vi "MoD Main-Optimize - Raman PK.vi"() -> ()   [LabVIEW 2015]
uses:
  <vilib>/silver_ctls/ArrayMatrixCluster/Real Matrix NI_Silver.ctl
  <vilib>/ni845x/ni845x.llb/ni845xControl.ctl
  <vilib>/MakerHub/LINX/Public/Peripherals/Analog/Analog Read 1 Chan.vi
  <vilib>/MakerHub/LINX/Public/Peripherals/Analog/Analog Read N Chans.vi
  <vilib>/MakerHub/LINX/Private/Local IO/LinxAnalogRead.vi
  <vilib>/MakerHub/LINX/Public/Utilities/Check Channel.vi
  <vilib>/addons/control/pid/pid.llb/PID Control Input Filter (DBL).vi
  <vilib>/MakerHub/LINX/Private/Utilties/Generate Error.vi
  <vilib>/addons/control/pid/autopid.llb/PID Online Autotuning (Relay Feedback).vi
  <vilib>/Analysis/Matrix/Numeric/Conversions/Array To Matrix - RA2.vi
  <vilib>/ni845x/ni845x.llb/NI-845x Close Device Reference.vi
  <vilib>/addons/control/pid/NI_PID_autopid.lvlib
  <vilib>/addons/control/pid/NI_PID_pid.lvlib
  <vilib>/Analysis/Matrix/NI_Matrix.lvlib
  <vilib>/MakerHub/LINX/LMH-LINX.lvlib
  <instrlib>/Harvard Apparatus PHD Ultra Series/Harvard Apparatus PHD Ultra Series.lvlib
panel:
  out "running?":bool=TRUE
  out "new_reactor_volume":bool[](array[boolean])
  out "new_reactor_length":bool[](array[boolean])
  out "Phase_Sensor_voltage":dbl
  out "P_tot":dbl
  out "pause for ms":bool=TRUE
  out "stop_xl_write":bool=TRUE
  out "Num_exp_till_pause":i32
  out "Syringe_pump?":bool=TRUE
  out "System Error":bool=TRUE
  out "error out":errorcluster
  out "Pump setpoint(ul/min) 6":dbl format="%#_13g"
  out "Pump setpoint(ul/min) 5":dbl format="%#_13g"
  out "Pump setpoint(ul/min) 4":dbl format="%#_13g"
  out "Pump setpoint(ul/min) 3":dbl format="%#_13g"
  out "Pump setpoint(ul/min) 2":dbl format="%#_13g"
  out "Pump setpoint(ul/min) 1":dbl format="%#_13g"
  out "Volume (ul) 5":dbl format="%#_13g"
  out "Volume (ul) 4":dbl format="%#_13g"
  out "Volume (ul) 3":dbl format="%#_13g"
  out "Volume (ul) 2":dbl format="%#_13g"
  out "Volume (ul) 1":dbl format="%#_13g"
  in  "tau 5":dbl format="%#_13g"
  out "tau 4":dbl format="%#_13g"
  out "tau 3":dbl format="%#_13g"
  out "tau 2":dbl format="%#_13g"
  out "tau 1":dbl format="%#_13g"
  out "Reactor Length":dbl format="%#_13g"
  out "Flowrate Sensor 2":dbl format="%#_13g"
  out "Flowrate Sensor 1":dbl format="%#_13g"
  out "Pressure 2":dbl format="%#_13g"
  out "Pressure 1":dbl format="%#_13g"
  out "Temperature Control 5":bool=TRUE
  out "Temperature Control 4":bool=TRUE
  out "Temperature Control 3":bool=TRUE
  out "Temperature Control 2":bool=TRUE
  out "Temperature Control 1":bool=TRUE
  out "Temperature SP 5":dbl format="%#_g'C"
  out "Temperature SP 4":dbl format="%#_g'C"
  out "Temperature SP 3":dbl format="%#_g'C"
  out "Temperature SP 2":dbl format="%#_g'C"
  out "Temperature SP 1":dbl format="%#_g'C"
  in  "Bay Temperature 5":dbl
  in  "SSR Duration 5":dbl
  in  "SSR Duration 4":dbl
  in  "SSR Duration 3":dbl
  in  "SSR Duration 2":dbl
  in  "SSR Duration 1":dbl
  in  "Total Product Amount":dbl=1.0 format="%#_gml"
  out "Setup Error":bool=TRUE
  out "Error Message":string
  out "ID CTR":i32
  in  "Tab Control":T1(tab)
  out "Reagent pic 5":picture
  in  "reagent name 5":string
  out "Reagent Pic 4":picture
  in  "reagent name 4":string=" 2,5-hexanedione"
  out "Reagent Pic 3":picture
  in  "reagent  name 3":string
  in  "Product name":string
  in  "reagent name 1":string="2,5-hexanedione"
  out "Reagent Pic 1":picture
  in  "Vr5":dbl format="%#_guL"
  in  "Vr4":dbl format="%#_guL"
  in  "Vr3":dbl format="%#_guL"
  in  "Vr2":dbl format="%#_guL"
  in  "Vr1":dbl format="%#_guL"
  in  "System decide help Button":bool
  in  "Reaction Scheme Confirm":bool
  in  "Synthesis Route Array":string[][](array[string])=[["Hexanedione", "1", "PhB(OH)2", "", "", ""], ["ethanolamine", "1", "-", "-", "-", "-"], ["", "", "-", "-", "-", "-"], ["", "", "-", "-", "-", "-"], ["", "", "-", "-", "-", "-"], ["", "", "-", "-", "-", "-"]]
  in  "System decide help Button 2":bool
  out "Setup Confirm":bool=TRUE
  in  "BAY 1":u16(ring) items=["               Bypass", "         Heated Reactor", "    Small Heated Reator", "         Cooled Reactor", "      Packed Bed Reactor", "          Photo Reactor", "             Separator"]
  in  "BAY 5":u16(ring) items=["               Bypass", "         Heated Reactor", "    Small Heated Reactor", "         Cooled Reactor", "     Packed Bed Reactor", "         Photo Reactor", "             Separator"]
  in  "BAY 4":u16(ring) items=["                Bypass", "         Heated Reactor", "    Small Heated Reactor", "         Cooled Reactor", "     Packed Bed Reactor", "         Photo Reactor", "             Separator"]
  in  "BAY 3":u16(ring)=2 items=["               Bypass", "         Heated Reactor", "    Small Heated Reactor", "         Cooled Reactor", "     Packed Bed Reactor", "          Photo Reactor", "             Separator"]
  in  "BAY 2":u16(ring) items=["               Bypass", "         Heated Reactor", "    Small Heated Reactor", "         Cooled Reactor", "      Packed Bed Reactor", "          Photo Reactor", "             Separator"]
  out "Reagent Pic 2":picture
  out "Product Pic":picture
  in  "reagent name 2":string="ethanolamine"
  in  "reagent name 6":string
  out "Reagent Pic 6":picture
  in  "System Parameters Help Button":bool
  out "Setup Confirm 2":bool
  in  "System Parameters Confirm Button":bool
  in  "Bay Parameters":T2={"Bay 1 "={"Pump 1 Flowrate"=0.0, "optimize_temp"=FALSE, "optimize_tau"=FALSE, "Run at set flowrate"=FALSE, "Pump 2 Flowrate"=0.0, "Temperature Params"=[40.0, 100.0, 100.0], "pump params 1"=[57.0, 122.0, 325.0], "pump params 2"=[57.0, 122.0, 325.0], "Temperature"=0.0, "Run at set temperature"=FALSE}, "Bay 2 "={"Pump 3 Flowrate"=0.0, "optimize_temp"=FALSE, "optimize_tau"=FALSE, "Run at set flowrate"=FALSE, "Temperature Params"=[40.0, 100.0, 100.0], "Resisdence time params"=[1.0, 5.0, 650.0], "pump_at_ratio"=FALSE, "pump_num_ratio"=4.0, "Temperature"=0.0, "Run at set temperature"=FALSE}, "Bay 3 "={"Pump 4 Flowrate"=100.0, "optimize_temp"=TRUE, "optimize_tau"=TRUE, "Run at set flowrate"=FALSE, "Temperature Params"=[40.0, 80.0, 100.0], "Resisdence time params"=[40.0, 401.0, 0.0], "pump_at_ratio"=FALSE, "pump_num_ratio"=0.05, "Temperature "=0.0, "Run at set temperature"=FALSE}, "Bay 4 "={"Pump 5 Flowrate"=40.0, "Run at set flowrate"=FALSE, "optimize_temp"=FALSE, "optimize_tau"=FALSE, "Resisdence time params"=[40.6, 406.0, 225.0], "Temperature Params"=[40.0, 100.0, 80.0], "pump_at_ratio"=FALSE, "pump_num_ratio"=1.0, "Temperature"=0.0, "Run at set temperature"=FALSE}, "Bay 5 "={"Pump 6 Flowrate"=0.0, "Run at set flowrate"=FALSE, "optimize_temp"=FALSE, "optimize_tau"=FALSE, "Resisdence time params"=[7.62, 114.27, 0.0], "Temperature Params"=[0.0, 0.0, 0.0], "pump_at_ratio"=FALSE, "pump_num_ratio"=0.5, "Temperature"=0.0, "Run at set temperature"=FALSE}, "Excel File Name"="C:\\Users\\HPLC\\Dropbox (MIT)\\MoD Files\\Data\\PK_Raman08302017", "Raman File Name"="\\\\Desktop-ld0eu12\\c\\Data\\MoD\\Paal_Knorr", "Matlab File"="C:\\Users\\HPLC\\Dropbox (MIT)\\MoD Files\\Data\\PK_Raman08302017_1", "Syringe for Pump 2?"=FALSE, "Num_conditons_per_wait"=2.0, "Continue from previous optimization?"=FALSE, "Total Number of Experiments 2"=12.0, "Hplc Wait time(min)"=8.0, "increas_decrease_hplc_peak"=TRUE, "Internal Standard?"=TRUE, "ISTD start"=3.0, "ISTD end"=4.0, "hplc_start"=6.0, "hplc_end"=7.0, "throughput_yield"=FALSE} {"Hplc Wait time(min)" format="%#_13g"; "Bay 5"."Temperature Params" format="%#_g'C"; "Bay 4"."Temperature Params" format="%#_g'C"; "Bay 3"."Temperature Params" format="%#_g'C"; "Bay 2"."Temperature Params" format="%#_g'C"; "Bay 1"."Temperature Params" format="%#_g'C"}
  out "System Confirm Not Clicked":string
  out "best_exp_num":dbl=1.0
  out "temperature_best":dbl[](array[numeric])
  out "Flowrates(ul/min)_best":dbl[](array[numeric])
  out "System Status":u16(ring)=2 caption="Sy" items=["System  Error", "System Running", "System Standby"]
  out "Current Experiment":dbl=1.0
  out "Total Number of Experiments":dbl=33.0
  out "Phase Sensor Chart":T3(graph)
  out "HPLC Analysis":bool
  out "Equlibrating Temperature":bool
  out "Flushing System":bool
  out "Calculate condition":bool
  out "Temperature 5":dbl format="%#_g'C"
  out "Temperature 4":dbl format="%#_g'C"
  out "Temperature 3":dbl format="%#_g'C"
  out "Temperature 2":dbl format="%#_g'C"
  out "Temperature 1":dbl format="%#_g'C"
  out "Flowrate Chart":T4(graph)
  out "Teperature Chart":T3(graph)
  out "Pump Setpoints Chart":T3(graph)
  out "Pressure Chart":T3(graph)
  out "Optimization_loop_index":i32
  out "curr_wait_time":dbl
  out "total_flush_time":dbl
  out "Temp SS? 5":bool=TRUE
  out "Temp SS? 4":bool=TRUE
  out "Temp SS? 3":bool=TRUE
  out "Temp SS? 2":bool=TRUE
  out "Temp SS? 1":bool=TRUE
  out "System Flushed?":bool
  out "stop_button clicked":bool
  out "experiment history":T5
  in  "Number of System Flushes per condtion":dbl=2.5
  in  "calculate volume 3":bool=TRUE
  in  "calculate volume 2":bool=TRUE
  in  "calculate volume 1":bool=TRUE
  in  "calculate volume 4":bool
  in  "calculate volume 5":bool
  in  "Extra system dead volume":dbl format="%#_gul"
  in  "new reactor length? 1":bool
  in  "tube_length(in)":dbl[](array[numeric])=[188.0, 188.0, 10.0, 10.0, 10.0]
  out "Pause Before Analysis":bool
  out "Chiller COMM Port":bool
  out "Arduino COMM Port 2":bool
  out "Temperature Sensor COMM Port":bool
  out "Flow Rate":bool
  out "Pressure":bool
  out "Pump COMM Port":bool
  in  "COMM Port :: Milligat Pumps":refnum<visa-resource-name>="COM10"
  in  "Arduino COMM Port":refnum<visa-resource-name>="COM3"
  in  "Sample Valve COMM::Port":refnum<visa-resource-name>="COM4"
  in  "COMM Port:: Harvard Syringe Pump":refnum<visa-resource-name>="COM5"
  in  "tube_id(in)":enum16{".01", ".02", ".03", ".04"}[](array[ring])=[enum.".03", enum.".03", enum.".03", enum.".03", enum.".03"]
  out "Total System Resisdence Time(min)":dbl
  in  "Debug_run_button":bool
  in  "new reactor length? 2":bool
  in  "new reactor length? 3":bool
  in  "new reactor length? 4":bool
  in  "new reactor length? 5":bool
  in  "IR Sensor Device":T6="USB0::0x3923::0x7514::01B3FF21::RAW"
  out "Stop":bool=TRUE
  in  "Run_Stop_cluster":T7
  # "Molecules on Demand"
  # "Synthetic Route"
  # "5"
  # "6"
  # "4"
  # "Product"
  # "1"
  # "2"
  # "3"
  # "Reagent List"
  # "Concentration(M)"
  # "Molecule"
  # "1"
  # "1"
  # "2"
  # "2"
  # "3"
  # "3"
  # "4"
  # "4"
  # "5"
  # "6"
  # "5"
  # "6"
  # "Product"
  # "Reactor Volume:"
  # "Optimization Parameters"
  # "Pause after"
  # "Experiments"
  # "Optimize for"
  # "to"
  # "of HPLC Peak from"
  # "from"
  # "to"
  # "min"
  # "min"
  # "HPLC runtime"
  # "# Iterations"
  # "Reporting"
  # "Excel Output File Name"
  # "Raman File Path"
  # "MATLAB File Path"
  # "Temperature"
  # "Flowrate(ul/min)"
  # "Lower Bound"
  # "Upper Bound"
  # "Optimize?"
  # "-or-"
  # "Run at"
  # "times incoming flow"
  # "Setpoint"
  # "Temperature"
  # "Flowrate(ul/min)"
  # "Lower Bound"
  # "Upper Bound"
  # "Optimize?"
  # "-or-"
  # "Run at"
  # "times incoming flow"
  # "Setpoint"
  # "Temperature"
  # "Flowrate(ul/min)"
  # "Lower Bound"
  # "Upper Bound"
  # "Optimize?"
  # "-or-"
  # "Run at"
  # "times incoming flow"
  # "Setpoint"
  # "Temperature"
  # "Flowrate 3 (ul/min)"
  # "Lower Bound"
  # "Upper Bound"
  # "Optimize?"
  # "-or-"
  # "Run at"
  # "times incoming flow"
  # "Setpoint"
  # "Temperature"
  # "Flowrate 1(ul/min)"
  # "Flowrate 2(ul/min)"
  # "Lower Bound"
  # "Upper Bound"
  # "Optimize?"
  # "Setpoint"
  # "Pressure (psi)"
  # "System Status"
  # "Temperature('C)"
  # "BAY"
  # "1"
  # "2"
  # "3"
  # "4"
  # "5"
  # "Pump Flowrate Setpoint(ul/min)"
  # "Flowrate (ul/min)"
  # "Phase Sensor"
  # "Current Experiment"
  # "Temperature('C)"
  # "Flowrate(ul/min)"
  # "Exp"
  # "Current Best Condition"
  # "Time to reach steady state:"
  # "Current Wait Time:"
  # "Experimental Steps"
  # "Calculated New Conditions"
  # "Steady State"
  # "Analyzed Raman"
  # "Equilibrated Temperature"
  # "Tube Length (cm)"
  # "Bay"
  # "Tube ID (in)"
  # "Calculate Volume"
  # "Use new tube length"
  # "1."
  # "2."
  # "3."
  # "4."
  # "5."
  # "Reactor Lengths\n*Heated Reactor - 188cm * Small Reactor - 99cm * Bypass - 10cm * Separator - *"
  # "All Experimental Data"
  # "P1"
  # "P2"
  # "P3"
  # "P4"
  # "P5"
  # "P6"
  # "T1"
  # "T2"
  # "T3"
  # "T4"
  # "T5"
  # "Obj_fun"
  # "HPLC_Data"
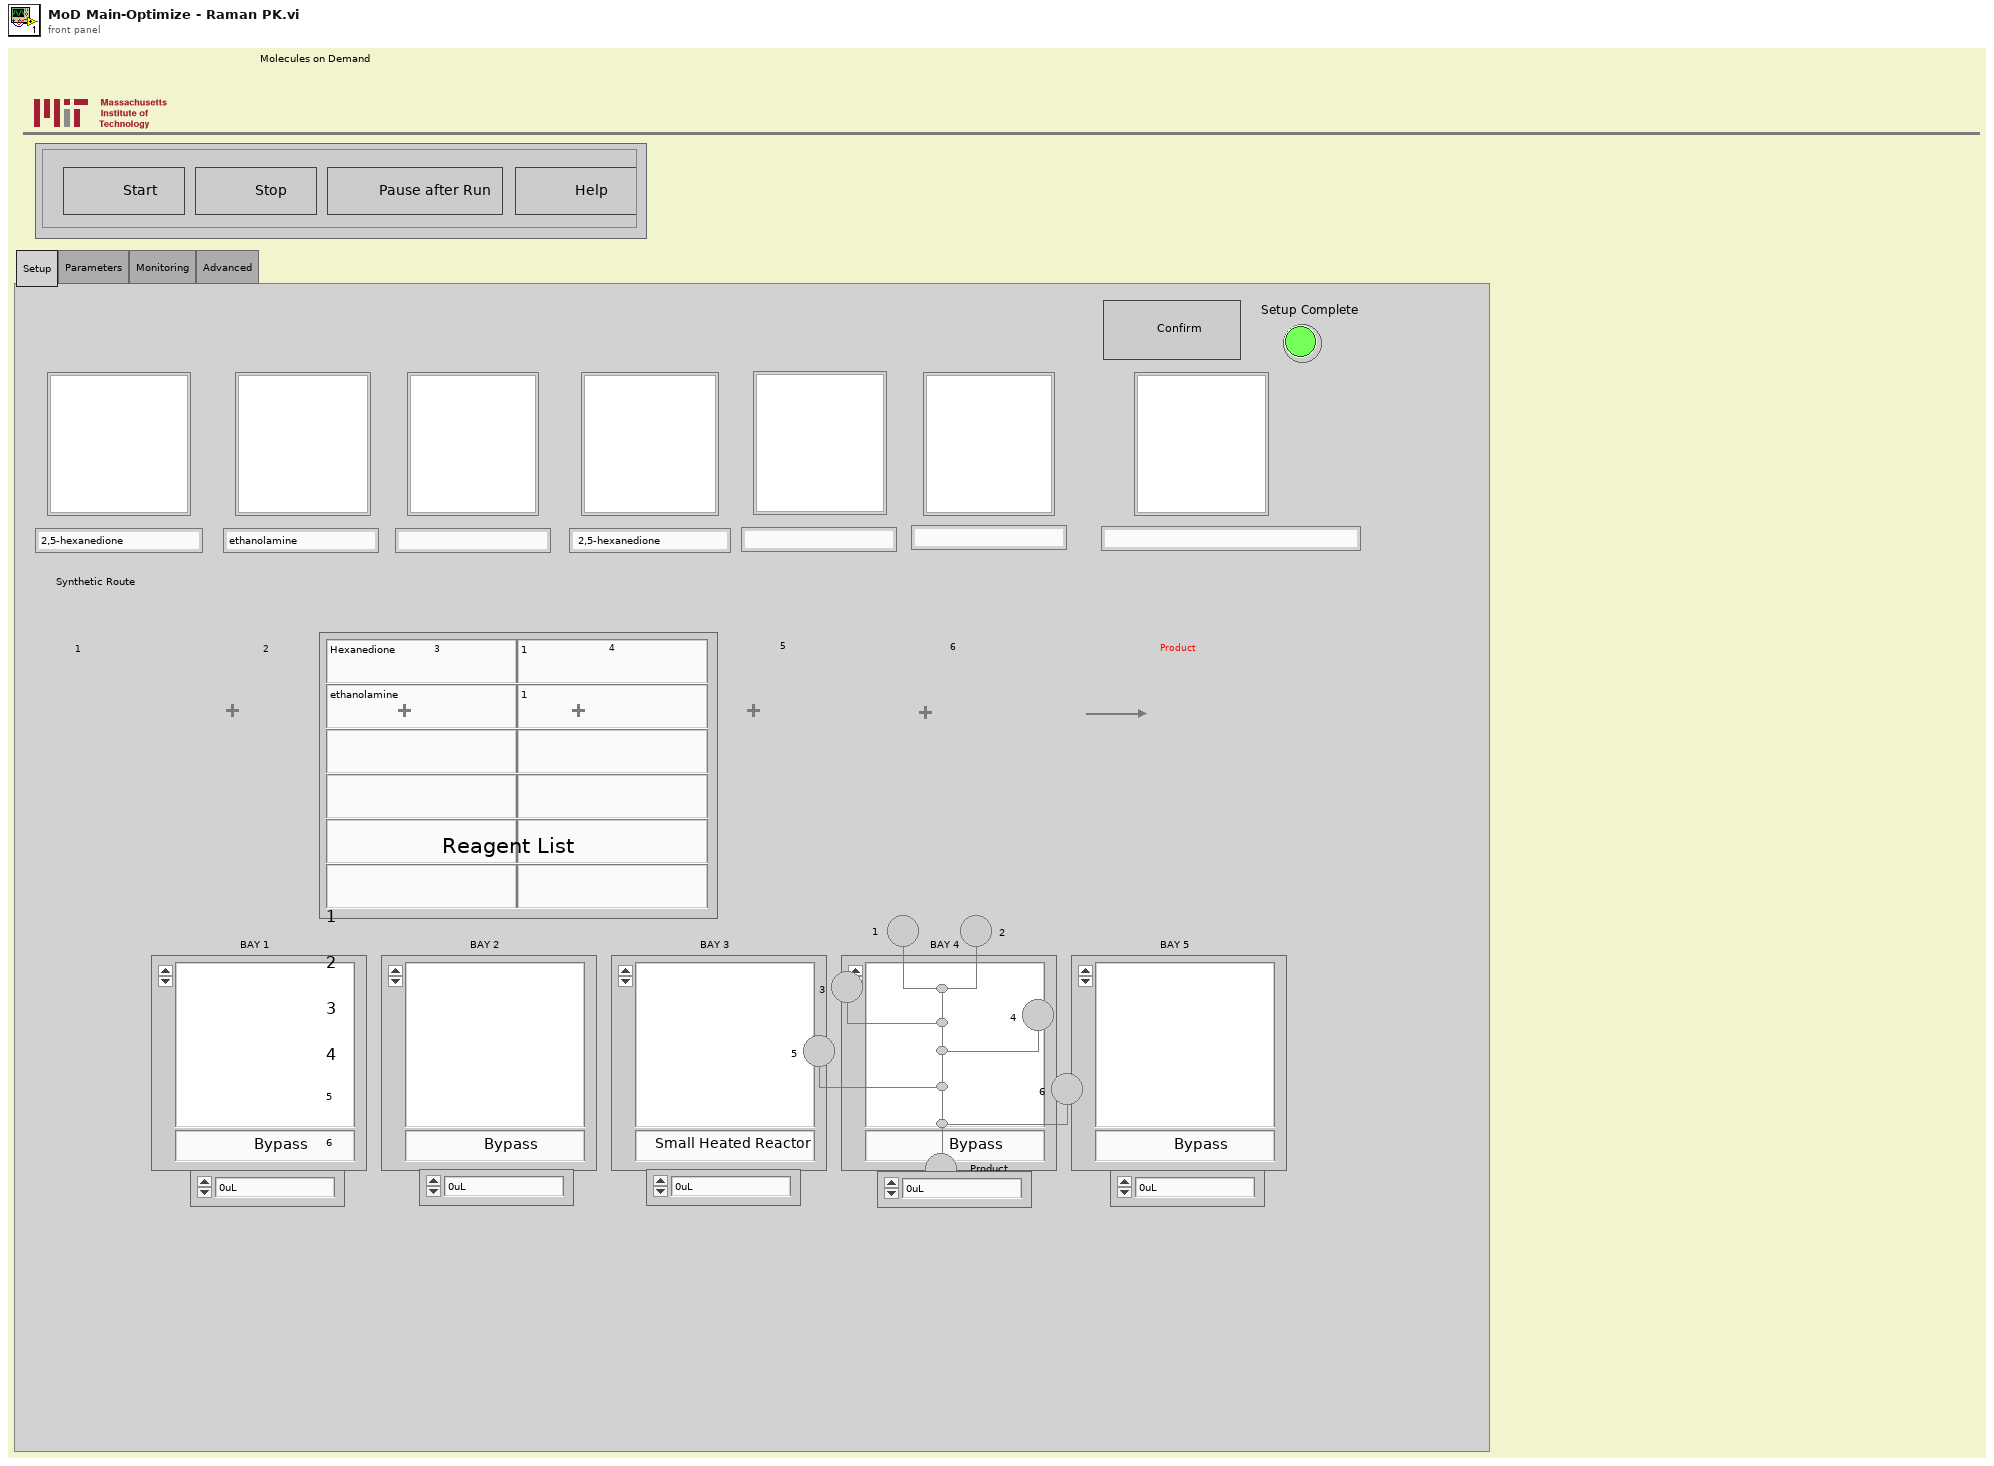
[diagram p1: front panel]
types:
  T1 = enum32{"Setup", "Parameters", "Monitoring", "Advanced"}
  T2 = cluster{"Bay 1 ":cluster{"Pump 1 Flowrate":dbl, "optimize_temp":bool, "optimize_tau":bool, "Run at set flowrate":bool, "Pump 2 Flowrate":dbl, "Temperature Params":dbl[], "pump params 1":dbl[], "pump params 2":dbl[], "Temperature":dbl, "Run at set temperature":bool}, "Bay 2 ":cluster{"Pump 3 Flowrate":dbl, "optimize_temp":bool, "optimize_tau":bool, "Run at set flowrate":bool, "Temperature Params":dbl[], "Resisdence time params":dbl[], "pump_at_ratio":bool, "pump_num_ratio":dbl, "Temperature":dbl, "Run at set temperature":bool}, "Bay 3 ":cluster{"Pump 4 Flowrate":dbl, "optimize_temp":bool, "optimize_tau":bool, "Run at set flowrate":bool, "Temperature Params":dbl[], "Resisdence time params":dbl[], "pump_at_ratio":bool, "pump_num_ratio":dbl, "Temperature ":dbl, "Run at set temperature":bool}, "Bay 4 ":cluster{"Pump 5 Flowrate":dbl, "Run at set flowrate":bool, "optimize_temp":bool, "optimize_tau":bool, "Resisdence time params":dbl[], "Temperature Params":dbl[], "pump_at_ratio":bool, "pump_num_ratio":dbl, "Temperature":dbl, "Run at set temperature":bool}, "Bay 5 ":cluster{"Pump 6 Flowrate":dbl, "Run at set flowrate":bool, "optimize_temp":bool, "optimize_tau":bool, "Resisdence time params":dbl[], "Temperature Params":dbl[], "pump_at_ratio":bool, "pump_num_ratio":dbl, "Temperature":dbl, "Run at set temperature":bool}, "Excel File Name":string, "Raman File Name":string, "Matlab File":string, "Syringe for Pump 2?":bool, "Num_conditons_per_wait":dbl, "Continue from previous optimization?":bool, "Total Number of Experiments 2":dbl, "Hplc Wait time(min)":dbl, "increas_decrease_hplc_peak":bool, "Internal Standard?":bool, "ISTD start":dbl, "ISTD end":dbl, "hplc_start":dbl, "hplc_end":dbl, "throughput_yield":bool}
  T3 = cluster{"[0]":dbl, "[1]":dbl, "[2]":dbl, "[3]":dbl, "[4]":dbl, "[5]":dbl, "[6]":dbl, "[7]":dbl, "[8]":dbl}
  T4 = cluster{"[0]":i32, "[1]":i32, "[2]":i32, "[3]":i32, "[4]":i32, "[5]":i32, "[6]":i32, "[7]":i32, "[8]":i32}
  T5 = typedef "Real Matrix NI_Silver.ctl" = dbl[][]
  T6 = typedef "ni845xControl.ctl" = refnum<k21>
  T7 = cluster{"Stop":bool, "Run":bool, "Stop Run Button":bool, "Help Button":bool}
  T8 = cluster{"Proportional gain Kc":dbl, "Integral time Ti (sec)":dbl, "Derivative time Ti (sec)":dbl}
  T9 = cluster{"type of controller":enum16{"P", "PI", "PID"}, "relay cycles":i32, "relay amplitude":dbl, "control specifications":enum16{"Fast", "Normal", "Slow"}, "PV noise level":dbl}
  T10 = typedef "LMH-LINX.lvlib/LINX Ref.ctl" = cluster{"IO":T11, "Interface":T12, "LINX Device Config":T13}
  T11 = typedef "LMH-LINX.lvlib/Platform.ctl" = enum16{"Remote", "Local"}
  T12 = typedef "LMH-LINX.lvlib/Interface.ctl" = enum16{"Serial", "TCP"}
  T13 = typedef "LMH-LINX.lvlib/Device.lvlib/LINX Device Config.ctl" = cluster{"Interface":T12, "COM Port":refnum<visa-resource-name>, "TCP Configuration":T14, "Device Family":u8, "Device ID":u8, "Device Name":string, "TCP Ref":refnum<k5>, "Channels":T15}
  T14 = typedef "LMH-LINX.lvlib/Device.lvlib/TCP Config.ctl" = cluster{"IP Address":string, "Port":u16}
  T15 = typedef "LMH-LINX.lvlib/Channels.ctl" = cluster{"DI":u8[], "DO":u8[], "AI":u8[], "AO":u8[], "PWM":u8[], "QE":u8[], "UART":u8[], "I2C 2":u8[], "SPI":u8[], "CAN":u8[], "Servo":u8[], "AI Ref (V)":dbl, "AI Resolution (Bits)":u8, "AO Ref (V)":dbl, "AO Resolution (Bits)":u8}
  T16 = typedef "imagedata.ctl" = cluster{"image type":i32, "image depth":i32, "image":u8[], "mask":u8[], "colors":u32[], "Rectangle":cluster{"left":i16, "top":i16, "right":i16, "bottom":i16}}
  T17 = cluster{"proportional gain (Kc)":dbl, "integral time (Ti, min)":dbl, "derivative time (Td, min)":dbl}
  T18 = typedef "NI_Matrix.lvlib/RealMatrix.ctl" = dbl[][]
  T19 = enum16{"Left Button", "Center Button", "Right Button", "Window Close"}
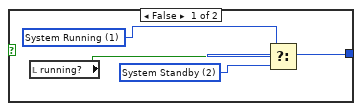
[diagram p3: hidden frame]
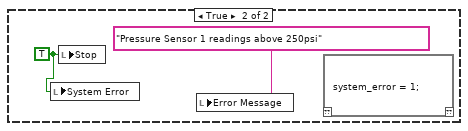
[diagram p5: hidden frame]
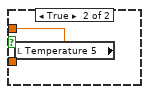
[diagram p6: hidden frame]
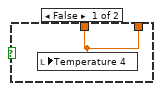
[diagram p7: hidden frame]
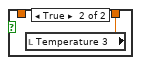
[diagram p8: hidden frame]
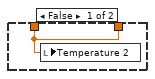
[diagram p9: hidden frame]
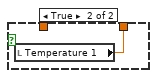
[diagram p10: hidden frame]
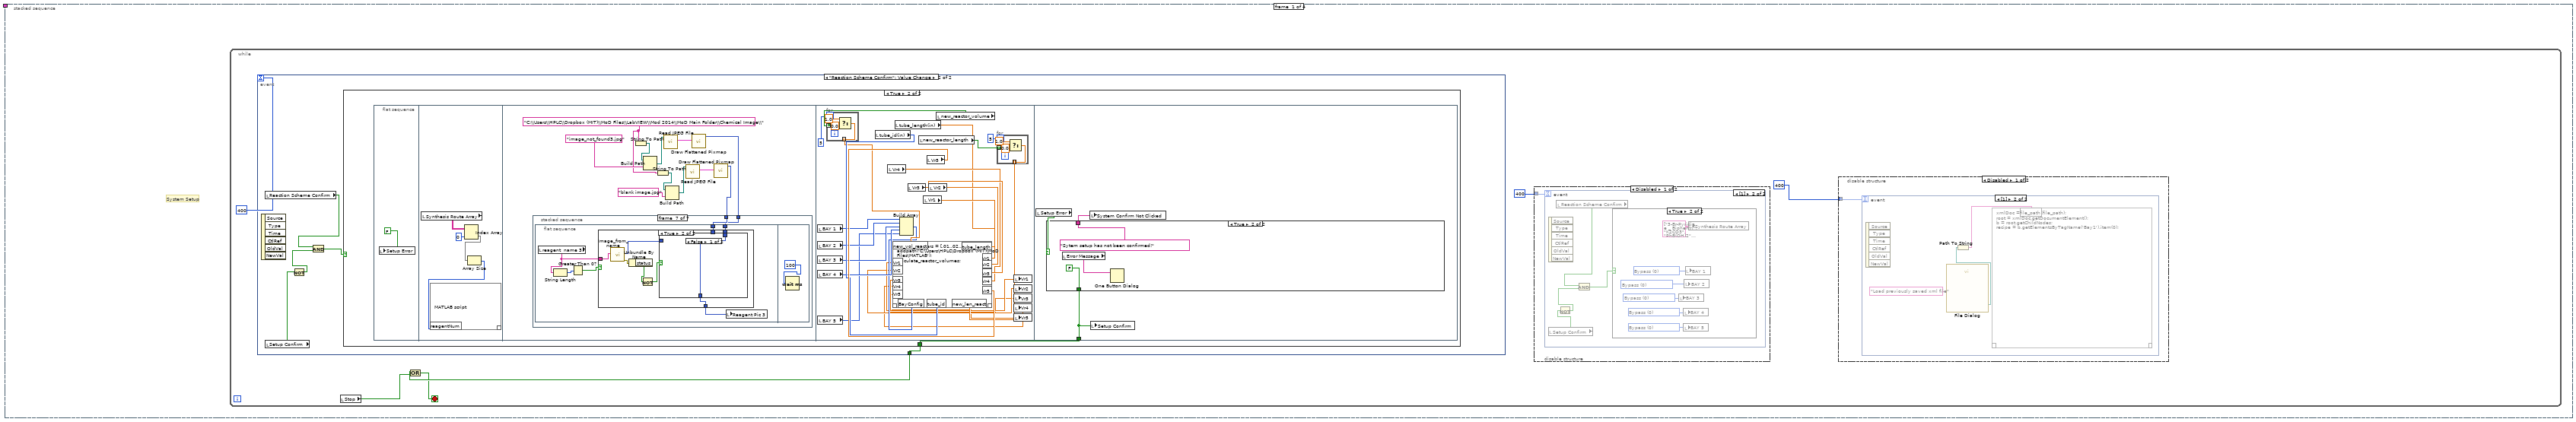
[diagram p11: hidden frame]
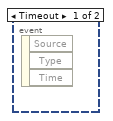
[diagram p12: hidden frame]
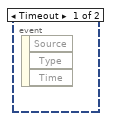
[diagram p14: hidden frame]
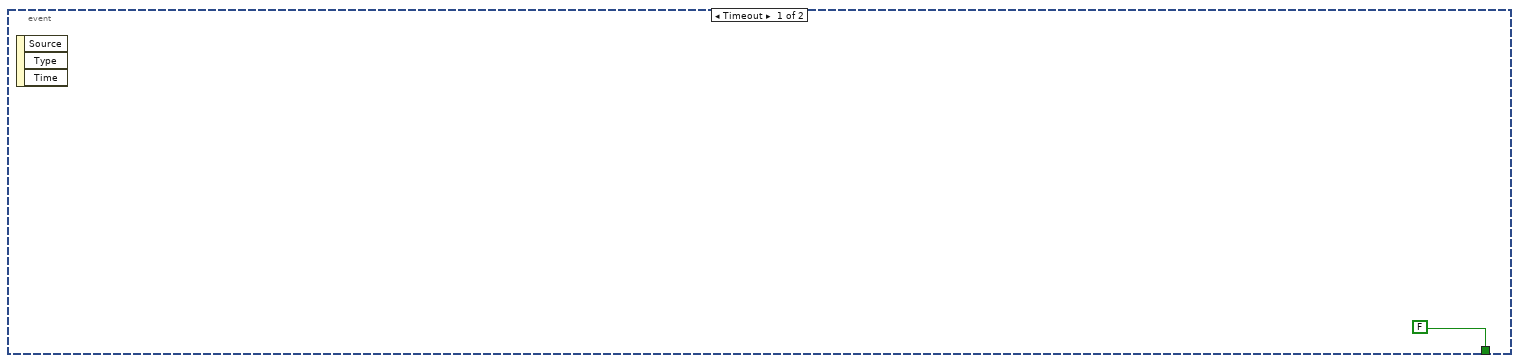
[diagram p17: hidden frame]
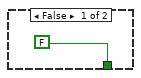
[diagram p18: hidden frame]
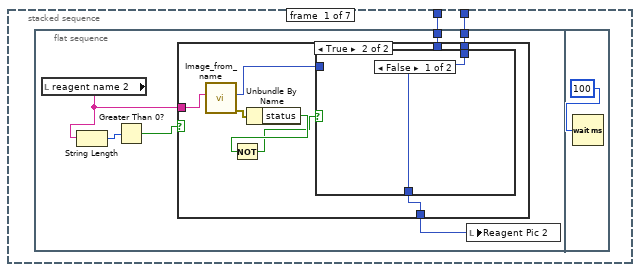
[diagram p19: hidden frame]
diagram:
  # "Assume User always uses the first bay first"
  n1 = flat-sequence {
    tunnel: ["COMM Port :: Milligat Pumps"] -> w9
    tunnel: ["Arduino COMM Port"] -> w8
    tunnel: [w11] -> w5
    tunnel: ["Bay Parameters"] -> w4
    tunnel: [w60] -> w10
    tunnel: w9 -> [w60]
    tunnel: w8 -> [w48]
    tunnel: [w54] -> w7
    tunnel: [w52] -> w6
    tunnel: w5 -> [w52]
    tunnel: w4 -> [w50]
    tunnel: [w47] -> w3
    tunnel: w10 -> [w66]
    tunnel: w7 -> [w65]
    tunnel: w6 -> [w63]
    tunnel: w3 -> [w61]
    tunnel: [w61] -> w1
    tunnel: [w1314] -> w2
    tunnel: w1 -> [w1314]
    tunnel: w2 -> [w1315]
    frame #0 {
      w36 = FALSE ("Equlibrating Temperature")
      n2 = script code="TempArr1=[23 23 23 23 23 23 23 23 23 23]';\nTempArr2=[23 23 23 23 23 23 23 23 23 23]';\nTempArr3=[23 23 23 23 23 23 23 23 23 23]';\nTempArr4=[23 23 23 23 23 23 23 23 23 23]';\nTempArr5=[23 23 23 23 23 23 23 23 23 23]';\nTempArrLED=[23 23 23 23 23 23 23 23 23 23]';\ntemp_error1 =0;\ntemp_error2 =0;\ntemp_error3 =0;\ntemp_error4 =0;\ntemp_error5 =0;\ntemp_check1 = 0;\ntemp_check2 = 0;\ntemp_check3 = 0;\ntemp_check4 = 0;\ntemp_check5 = 0;\nT1=23;\nT2=23;\nT3=23;\nT4=23;\nT5=23;"() -> ()  [unwired: 1 in, 1 out]
      n3 = Build Array("calculate volume 1", "calculate volume 2", "calculate volume 3", "calculate volume 4", "calculate volume 5") -> (→"new_reactor_volume":bool[])
      n4 = Build Array("new reactor length? 1", "new reactor length? 2", "new reactor length? 3", "new reactor length? 4", "new reactor length? 5") -> (→"new_reactor_length":bool[])
      n5 = call <vilib>:"Initialize.vi"("VISA resource name"="COMM Port:: Harvard Syringe Pump") -> ("VISA resource name out"=w11:refnum<visa-resource-name>)  [unwired: 9 in, 1 out]
      "Stop" <- FALSE ("Stop")
      "ID CTR" <- 0
      "Setup Confirm" <- FALSE ("Setup Confirm")
      "Error Message" <- "System shutdown sucessfully. No errors to report." ("Error Message")
      "Setup Error" <- FALSE ("Setup Error")
      "Reactor Length" <- 10.5
      "System Error" <- FALSE ("System Error")
      "Num_exp_till_pause" <- 0 ("Num_exp_till_pause")
      "Equlibrating Temperature" <- w36
      "Calculate condition" <- w36
      "Flushing System" <- w36
      "HPLC Analysis" <- w36
      "stop_xl_write" <- FALSE ("stop_xl_write")
      "Pump setpoint(ul/min) 1" <- 0.0 ("Pump setpoint(ul/min) 1")
      "Pump setpoint(ul/min) 2" <- 0.0 ("Pump setpoint(ul/min) 2")
      "Pump setpoint(ul/min) 4" <- 0.0 ("Pump setpoint(ul/min) 4")
      "Pump setpoint(ul/min) 6" <- 0.0 ("Pump setpoint(ul/min) 6")
      "Pump setpoint(ul/min) 3" <- 0.0 ("Pump setpoint(ul/min) 3")
      "Pump setpoint(ul/min) 5" <- 0.0 ("Pump setpoint(ul/min) 5")
      "pause for ms" <- FALSE ("pause for ms")
      "Setup Confirm 2" <- FALSE ("Setup Confirm 2")
      "running?" <- FALSE ("running?")
    }
    frame #1 {
      w49 = FALSE
      w59 = 23
      (unwired) path "C:/Users/User1/Documents/Lab/MoD/Images"
      n6 = disable-structure shown="Disabled" {
        frame Disabled {
          n7 = local read "BAY 2"() -> ()  [unwired: 1 out]
          n8 = local read "BAY 3"() -> ()  [unwired: 1 out]
          n9 = local read "BAY 4"() -> ()  [unwired: 1 out]
          n10 = local read "BAY 5"() -> ()  [unwired: 1 out]
          n11 = local read "BAY 1"() -> ()  [unwired: 1 out]
        }
        frame Enabled {
        }
      }
      n12 = local write "Debug_run_button"(TRUE) -> ()
      n13 = call <vilib>:"Initialize.vi"("Serial Port"=w48) -> ("LINX Resource"=w47:T10)  [unwired: 8 in, 2 out]
      n14 = local write "System Parameters Confirm Button"(w49) -> ()
      n15 = local write "Setup Confirm 2"(w49) -> ()
      n16 = Unbundle By Name(w50) -> ("Syringe for Pump 2?"=→"Syringe_pump?":bool)
      n17 = local write "Temperature 1"(w59) -> ()
      n18 = local write "Temperature 2"(w59) -> ()
      n19 = local write "Temperature 3"(w59) -> ()
      n20 = local write "Temperature 4"(w59) -> ()
      n21 = local write "Temperature 5"(w59) -> ()
      n22 = local write "Temperature SP 1"(w59) -> ()
      n23 = local write "Temperature SP 2"(w59) -> ()
      n24 = local write "Temperature SP 3"(w59) -> ()
      n25 = local write "Temperature SP 4"(w59) -> ()
      n26 = local write "Temperature SP 5"(w59) -> ()
      n27 = Current VI's Path() -> (path=w58:path)
      n28 = Strip Path(path=w58) -> (stripped path=w56:path)  [unwired: 1 out]
      n29 = Strip Path(path=w56) -> (stripped path=w55:path)  [unwired: 1 out]
      n30 = Build Path(base path=w55, name or relative path="MATLAB") -> (appended path=w54:path)
    }
    frame #2 {
      # "Main Help Dialog Popup"
      n31 = while {
        stop <- w1308 stop-if-true
        n32 = event shown="[6] \"Run_Stop_cluster.Run\": Value Change" {
          selector: _ -> [_ _ _ _ _ _ _]
          dyn-events: _ -> [_ _ _ _ _ _ _]
          timeout: 100 -> [_ _ _ _ _ _ _]
          event Timeout {
            n33 = event-data() -> ()  [unwired: 1 in, 3 out]
          }
          event "Run_Stop_cluster.Help Button": Value Change {
            n34 = local read "Run_Stop_cluster"() -> (w1311:T7)
            n35 = event-data() -> ()  [unwired: 1 in, 4 out]
            n36 = Unbundle By Name(w1311) -> ("Help Button"=w1310:bool)
            n37 = case shown="True" w1310 {
              frame False {
              }
              frame True {
                n38 = call "help.vi"() -> ()  [unwired: 11 in]
              }
            }
          }
          event "System decide help Button": Value Change {
            n39 = event-data() -> ()  [unwired: 1 in, 5 out]
            n40 = call "help_synthesis_man-auto_instructions.vi"() -> ()  [unwired: 12 in]
          }
          event "System Parameters Help Button": Value Change {
            n41 = event-data() -> ()  [unwired: 1 in, 5 out]
            n42 = call "help_parameters_setup.vi"() -> ()  [unwired: 12 in]
          }
          event "System decide help Button 2": Value Change {
            n43 = event-data() -> ()  [unwired: 1 in, 5 out]
            n44 = call "help_synthesis_route_instructions.vi"() -> ()  [unwired: 12 in]
          }
          event "Run_Stop_cluster.Stop": Value Change {
            n45 = event-data() -> ()  [unwired: 1 in, 5 out]
            n46 = local write "Stop"(TRUE) -> ()
          }
          event "Run_Stop_cluster.Run": Value Change {
            n47 = event-data() -> ()  [unwired: 1 in, 5 out]
            n48 = local write "running?"(TRUE) -> ()
          }
        }
        n49 = local read "Stop"() -> (w1308:bool)
      }
      n50 = stacked-sequence {
        tunnel: w66 -> [_ _ _ _]
        tunnel: w65 -> [_ w425 _ _]
        tunnel: w63 -> [_ _ _ w592]
        tunnel: w61 -> [_ _ _ w590]
        frame #0 {
          # "System Setup"
          n51 = while {
            stop <- w200 stop-if-true
            n52 = event shown="[1] \"Reaction Scheme Confirm\": Value Change" {
              selector: _ -> [_ _]
              dyn-events: _ -> [_ _]
              timeout: 400 -> [_ _]
              tunnel: [FALSE w220] -> w202
              event Timeout {
                n53 = event-data() -> ()  [unwired: 1 in, 3 out]
              }
              event "Reaction Scheme Confirm": Value Change {
                n54 = event-data() -> ()  [unwired: 1 in, 6 out]
                n55 = local read "Reaction Scheme Confirm"() -> (w224:bool)
                n56 = local read "Setup Confirm"() -> (w222:bool)
                n57 = Not(x=w222) -> (.not. x?=w221:bool)
                n58 = And(x=w224, y=w221) -> (x .and. y?=w223:bool)
                n59 = case shown="True" w223 {
                  tunnel: [FALSE w226] -> w220
                  frame False {
                  }
                  frame True {
                    n60 = flat-sequence {
                      tunnel: [w415] -> w226
                      frame #0 {
                        n61 = local write "Setup Error"(FALSE) -> ()
                      }
                      frame #1 {
                        n62 = local read "Synthesis Route Array"() -> (w230:string[][])
                        n63 = Index Array(array=w230, index (col)=0 ("disabled index (col)")) -> (element=w228:string[])  [unwired: 1 in]
                        n64 = Array Size(array=w228) -> (size(s)=w231:i32)
                        n65 = script code="MATLAB script"("reagentNum"=w231) -> ()  [unwired: 1 in, 1 out]
                      }
                      frame #2 {
                        w234 = "C:\\Users\\HPLC\\Dropbox (MIT)\\MoD Files\\LabVIEW\\Mod 2014\\MoD Main Folder\\Chemical Image\\" ("string")
                        n66 = String To Path(string=w234) -> (path=w240:path)
                        n67 = Build Path(base path=w240, name or relative path="image_not_found3.jpg") -> (appended path=w239:path)
                        n68 = String To Path(string=w234) -> (path=w237:path)
                        n69 = call <vilib>:"Read JPEG File.vi"("path to JPEG file"=w239) -> ("image data"=w242:T16)  [unwired: 1 in, 9 out]
                        n70 = Build Path(base path=w237, name or relative path="blank image.jpg") -> (appended path=w235:path)
                        n71 = call <vilib>:"Read JPEG File.vi"("path to JPEG file"=w235) -> ("image data"=w238:T16)  [unwired: 1 in, 9 out]
                        n72 = call <vilib>:"Draw Flattened Pixmap.vi"("image data"=w242) -> ("new picture"=w233:picture)  [unwired: 3 in, 5 out]
                        n73 = call <vilib>:"Draw Flattened Pixmap.vi"("image data"=w238) -> ("new picture"=w232:picture)  [unwired: 3 in, 5 out]
                        n74 = stacked-sequence {
                          tunnel: w233 -> [w244 w264 w284 w304 w324 w343 w363]
                          tunnel: w232 -> [w243 w263 w283 w303 w323 w344 w364]
                          frame #0 {
                            n75 = flat-sequence {
                              tunnel: w244 -> [w250]
                              tunnel: w243 -> [w248]
                              frame #0 {
                                n76 = local read "reagent name 2"() -> (w246:string)
                                n77 = String Length(string=w246) -> (length=w249:i32)
                                n78 = Greater Than 0?(x=w249) -> (x > 0?=w247:bool)
                                n79 = case shown="True" w247 {
                                tunnel: w250 -> [_ w256]
                                tunnel: w248 -> [w251 _]
                                tunnel: [w251 w255] -> w245
                                tunnel: w246 -> [_ w254]
                                frame False {
                                }
                                frame True {
                                n80 = call "Image_from_name.vi"("Chemical Name"=w254) -> ("error out"=w257:errorcluster, "Downloaded Picture"=w258:picture)  [unwired: 8 in, 1 out]
                                n81 = Unbundle By Name(w257) -> ("status"=w253:bool)
                                n82 = Not(x=w253) -> (.not. x?=w252:bool)
                                n83 = case shown="False" w252 {
                                tunnel: w258 -> [_ w261]
                                tunnel: [w259 w260] -> w255
                                tunnel: w256 -> [w259 _]
                                frame False {
                                }
                                frame True {
                                n84 = call <vilib>:"Draw Flattened Pixmap.vi"("picture"=w261) -> ("new picture"=w260:picture)  [unwired: 8 in]
                                }
                                }
                                }
                                }
                                n85 = local write "Reagent Pic 2"(w245) -> ()
                              }
                              frame #1 {
                                n86 = Wait (ms)(milliseconds to wait=100) -> ()  [unwired: 1 out]
                              }
                            }
                          }
                          frame #1 {
                            n87 = flat-sequence {
                              tunnel: w264 -> [w270]
                              tunnel: w263 -> [w268]
                              frame #0 {
                                n88 = local read "reagent name 1"() -> (w265:string)
                                n89 = String Length(string=w265) -> (length=w269:i32)
                                n90 = Greater Than 0?(x=w269) -> (x > 0?=w267:bool)
                                n91 = case shown="True" w267 {
                                tunnel: w270 -> [_ w276]
                                tunnel: w268 -> [w271 _]
                                tunnel: [w271 w275] -> w266
                                tunnel: w265 -> [_ w274]
                                frame False {
                                }
                                frame True {
                                n92 = call "Image_from_name.vi"("Chemical Name"=w274) -> ("error out"=w277:errorcluster, "Downloaded Picture"=w278:picture)  [unwired: 8 in, 1 out]
                                n93 = Unbundle By Name(w277) -> ("status"=w273:bool)
                                n94 = Not(x=w273) -> (.not. x?=w272:bool)
                                n95 = case shown="True" w272 {
                                tunnel: w278 -> [_ w281]
                                tunnel: [w279 w280] -> w275
                                tunnel: w276 -> [w279 _]
                                frame False {
                                }
                                frame True {
                                n96 = call <vilib>:"Draw Flattened Pixmap.vi"("picture"=w281) -> ("new picture"=w280:picture)  [unwired: 8 in]
                                }
                                }
                                }
                                }
                                n97 = local write "Reagent Pic 1"(w266) -> ()
                              }
                              frame #1 {
                                n98 = Wait (ms)(milliseconds to wait=100) -> ()  [unwired: 1 out]
                              }
                            }
                          }
                          frame #2 {
                            n99 = flat-sequence {
                              tunnel: w284 -> [w290]
                              tunnel: w283 -> [w288]
                              frame #0 {
                                n100 = local read "Product name"() -> (w285:string)
                                n101 = String Length(string=w285) -> (length=w289:i32)
                                n102 = Greater Than 0?(x=w289) -> (x > 0?=w287:bool)
                                n103 = case shown="True" w287 {
                                tunnel: w290 -> [_ w296]
                                tunnel: w288 -> [w291 _]
                                tunnel: [w291 w295] -> w286
                                tunnel: w285 -> [_ w294]
                                frame False {
                                }
                                frame True {
                                n104 = call "Image_from_name.vi"("Chemical Name"=w294) -> ("error out"=w297:errorcluster, "Downloaded Picture"=w298:picture)  [unwired: 8 in, 1 out]
                                n105 = Unbundle By Name(w297) -> ("status"=w292:bool)
                                n106 = Not(x=w292) -> (.not. x?=w293:bool)
                                n107 = case shown="False" w293 {
                                tunnel: w298 -> [_ w301]
                                tunnel: [w299 w300] -> w295
                                tunnel: w296 -> [w299 _]
                                frame False {
                                }
                                frame True {
                                n108 = call <vilib>:"Draw Flattened Pixmap.vi"("picture"=w301) -> ("new picture"=w300:picture)  [unwired: 8 in]
                                }
                                }
                                }
                                }
                                n109 = local write "Product Pic"(w286) -> ()
                              }
                              frame #1 {
                                n110 = Wait (ms)(milliseconds to wait=100) -> ()  [unwired: 1 out]
                              }
                            }
                          }
                          frame #3 {
                            n111 = flat-sequence {
                              tunnel: w304 -> [w310]
                              tunnel: w303 -> [w308]
                              frame #0 {
                                n112 = local read "reagent name 6"() -> (w305:string)
                                n113 = String Length(string=w305) -> (length=w309:i32)
                                n114 = Greater Than 0?(x=w309) -> (x > 0?=w307:bool)
                                n115 = case shown="True" w307 {
                                tunnel: w310 -> [_ w316]
                                tunnel: w308 -> [w311 _]
                                tunnel: [w311 w315] -> w306
                                tunnel: w305 -> [_ w314]
                                frame False {
                                }
                                frame True {
                                n116 = call "Image_from_name.vi"("Chemical Name"=w314) -> ("error out"=w317:errorcluster, "Downloaded Picture"=w318:picture)  [unwired: 8 in, 1 out]
                                n117 = Unbundle By Name(w317) -> ("status"=w312:bool)
                                n118 = Not(x=w312) -> (.not. x?=w313:bool)
                                n119 = case shown="False" w313 {
                                tunnel: w318 -> [_ w321]
                                tunnel: [w319 w320] -> w315
                                tunnel: w316 -> [w319 _]
                                frame False {
                                }
                                frame True {
                                n120 = call <vilib>:"Draw Flattened Pixmap.vi"("picture"=w321) -> ("new picture"=w320:picture)  [unwired: 8 in]
                                }
                                }
                                }
                                }
                                n121 = local write "Reagent Pic 6"(w306) -> ()
                              }
                              frame #1 {
                                n122 = Wait (ms)(milliseconds to wait=100) -> ()  [unwired: 1 out]
                              }
                            }
                          }
                          frame #4 {
                            n123 = flat-sequence {
                              tunnel: w324 -> [w330]
                              tunnel: w323 -> [w328]
                              frame #0 {
                                n124 = local read "reagent name 5"() -> (w325:string)
                                n125 = String Length(string=w325) -> (length=w329:i32)
                                n126 = Greater Than 0?(x=w329) -> (x > 0?=w327:bool)
                                n127 = case shown="True" w327 {
                                tunnel: w330 -> [_ w336]
                                tunnel: w328 -> [w331 _]
                                tunnel: [w331 w335] -> w326
                                tunnel: w325 -> [_ w334]
                                frame False {
                                }
                                frame True {
                                n128 = call "Image_from_name.vi"("Chemical Name"=w334) -> ("error out"=w337:errorcluster, "Downloaded Picture"=w338:picture)  [unwired: 8 in, 1 out]
                                n129 = Unbundle By Name(w337) -> ("status"=w332:bool)
                                n130 = Not(x=w332) -> (.not. x?=w333:bool)
                                n131 = case shown="False" w333 {
                                tunnel: w338 -> [_ w341]
                                tunnel: [w339 w340] -> w335
                                tunnel: w336 -> [w339 _]
                                frame False {
                                }
                                frame True {
                                n132 = call <vilib>:"Draw Flattened Pixmap.vi"("picture"=w341) -> ("new picture"=w340:picture)  [unwired: 8 in]
                                }
                                }
                                }
                                }
                                n133 = local write "Reagent pic 5"(w326) -> ()
                              }
                              frame #1 {
                                n134 = Wait (ms)(milliseconds to wait=100) -> ()  [unwired: 1 out]
                              }
                            }
                          }
                          frame #5 {
                            n135 = flat-sequence {
                              tunnel: w344 -> [w348]
                              tunnel: w343 -> [w347]
                              frame #0 {
                                n136 = local read "reagent name 4"() -> (w345:string)
                                n137 = String Length(string=w345) -> (length=w350:i32)
                                n138 = Greater Than 0?(x=w350) -> (x > 0?=w349:bool)
                                n139 = case shown="True" w349 {
                                tunnel: w347 -> [_ w356]
                                tunnel: w348 -> [w351 _]
                                tunnel: [w351 w355] -> w346
                                tunnel: w345 -> [_ w354]
                                frame False {
                                }
                                frame True {
                                n140 = call "Image_from_name.vi"("Chemical Name"=w354) -> ("error out"=w357:errorcluster, "Downloaded Picture"=w358:picture)  [unwired: 8 in, 1 out]
                                n141 = Unbundle By Name(w357) -> ("status"=w352:bool)
                                n142 = Not(x=w352) -> (.not. x?=w353:bool)
                                n143 = case shown="False" w353 {
                                tunnel: w358 -> [_ w361]
                                tunnel: [w359 w360] -> w355
                                tunnel: w356 -> [w359 _]
                                frame False {
                                }
                                frame True {
                                n144 = call <vilib>:"Draw Flattened Pixmap.vi"("picture"=w361) -> ("new picture"=w360:picture)  [unwired: 8 in]
                                }
                                }
                                }
                                }
                                n145 = local write "Reagent Pic 4"(w346) -> ()
                              }
                              frame #1 {
                                n146 = Wait (ms)(milliseconds to wait=100) -> ()  [unwired: 1 out]
                              }
                            }
                          }
                          frame #6 {
                            n147 = flat-sequence {
                              tunnel: w364 -> [w368]
                              tunnel: w363 -> [w367]
                              frame #0 {
                                n148 = local read "reagent  name 3"() -> (w365:string)
                                n149 = String Length(string=w365) -> (length=w370:i32)
                                n150 = Greater Than 0?(x=w370) -> (x > 0?=w369:bool)
                                n151 = case shown="True" w369 {
                                tunnel: w367 -> [_ w376]
                                tunnel: w368 -> [w371 _]
                                tunnel: [w371 w375] -> w366
                                tunnel: w365 -> [_ w374]
                                frame False {
                                }
                                frame True {
                                n152 = call "Image_from_name.vi"("Chemical Name"=w374) -> ("error out"=w377:errorcluster, "Downloaded Picture"=w378:picture)  [unwired: 8 in, 1 out]
                                n153 = Unbundle By Name(w377) -> ("status"=w372:bool)
                                n154 = Not(x=w372) -> (.not. x?=w373:bool)
                                n155 = case shown="False" w373 {
                                tunnel: w378 -> [_ w381]
                                tunnel: [w379 w380] -> w375
                                tunnel: w376 -> [w379 _]
                                frame False {
                                }
                                frame True {
                                n156 = call <vilib>:"Draw Flattened Pixmap.vi"("picture"=w381) -> ("new picture"=w380:picture)  [unwired: 8 in]
                                }
                                }
                                }
                                }
                                n157 = local write "Reagent Pic 3"(w366) -> ()
                              }
                              frame #1 {
                                n158 = Wait (ms)(milliseconds to wait=100) -> ()  [unwired: 1 out]
                              }
                            }
                          }
                        }
                      }
                      frame #3 {
                        n159 = local read "BAY 1"() -> (w393:u16)
                        n160 = local read "BAY 2"() -> (w392:u16)
                        n161 = local read "BAY 3"() -> (w391:u16)
                        n162 = local read "BAY 4"() -> (w390:u16)
                        n163 = local read "BAY 5"() -> (w389:u16)
                        n164 = local read "tube_id(in)"() -> (w400:enum16{".01", ".02", ".03", ".04"}[])
                        n165 = local read "Vr4"() -> (w403:dbl)
                        n166 = local read "tube_length(in)"() -> (w401:dbl[])
                        n167 = Build Array(w393, w392, w391, w390, w389) -> (w388:u16[])
                        n168 = local read "Vr3"() -> (w404:dbl)
                        n169 = local read "new_reactor_length"() -> (w398:bool[])
                        n170 = local read "Vr1"() -> (w406:dbl)
                        n171 = local read "Vr5"() -> (w402:dbl)
                        n172 = local read "Vr2"() -> (w405:dbl)
                        n173 = local read "new_reactor_volume"() -> (w396:bool[])
                        n174 = for {
                          N: 5 -> [_]
                          tunnel: w396 -> [w410] mode=indexing
                          tunnel: [w407] -> w394 mode=indexing
                          n175 = Select(t=1.0, s=w410, f=0.0) -> (s? t:f=w407:dbl)
                        }
                        n176 = for {
                          N: 5 -> [_]
                          tunnel: w398 -> [w414] mode=indexing
                          tunnel: [w411] -> w397 mode=indexing
                          n177 = Select(t=1.0, s=w414, f=0.0) -> (s? t:f=w411:dbl)
                        }
                        n178 = script code="tube_diameters = [.01,.02,.03,.04];\naddpath('C:\\Users\\HPLC\\Dropbox (MIT)\\MoD Files\\MATLAB');\ncalculate_reactor_volumes;"("BayConfig"=w388, "Vr1"=w406, "Vr2"=w405, "Vr3"=w404, "Vr4"=w403, "Vr5"=w402, "tube_length"=w401, "tube_id"=w400, "new_len_react"=w397, "new_vol_react"=w394) -> ("Vr1"=w387:dbl, "Vr2"=w386:dbl, "Vr3"=w385:dbl, "Vr4"=w384:dbl, "Vr5"=w383:dbl)  [unwired: 1 in, 1 out]
                        n179 = local write "Vr1"(w387) -> ()
                        n180 = local write "Vr2"(w386) -> ()
                        n181 = local write "Vr3"(w385) -> ()
                        n182 = local write "Vr4"(w384) -> ()
                        n183 = local write "Vr5"(w383) -> ()
                      }
                      frame #4 {
                        n184 = local read "Setup Error"() -> (w417:bool)
                        n185 = case shown="True" w417 {
                          tunnel: [TRUE FALSE] -> w415
                          tunnel: ["" "Sytem setup has not been confirmed!"] -> w416
                          frame False {
                          }
                          frame True {
                            n186 = local read "Error Message"() -> (w422:string)
                            n187 = One Button Dialog(message=w422) -> ()  [unwired: 1 in, 1 out]
                          }
                        }
                        n188 = local write "System Confirm Not Clicked"(w416) -> ()
                        n189 = local write "Setup Confirm"(w415) -> ()
                      }
                    }
                  }
                }
              }
            }
            n190 = local read "Stop"() -> (w201:bool)
            n191 = Or(x=w202, y=w201) -> (x .or. y?=w200:bool)
            n192 = disable-structure shown="Disabled" {
              disable-tunnel: 400 -> [w208 _]
              frame Disabled {
                n193 = event shown="[1]" {
                  selector: _ -> [_ _]
                  dyn-events: _ -> [_ _]
                  timeout: w208 -> [_ _]
                  event Timeout {
                    n194 = event-data() -> ()  [unwired: 1 in, 3 out]
                  }
                  event #1 (no event record) {
                    n195 = event-data() -> ()  [unwired: 1 in, 6 out]
                    n196 = local read "Setup Confirm"() -> (w209:bool)
                    n197 = local read "Reaction Scheme Confirm"() -> (w210:bool)
                    n198 = Not(x=w209) -> (.not. x?=w212:bool)
                    n199 = And(x=w210, y=w212) -> (x .and. y?=w211:bool)
                    n200 = case shown="True" w211 {
                      frame False {
                      }
                      frame True {
                        w214 = u16 0 items=["                     Bypass", "                Hot Reactor", "                 Separator"] ("BAY 5")
                        w215 = u16 0 items=["                     Bypass", "                Hot Reactor", "                  Separator"] ("BAY 4")
                        w216 = u16 0 items=["                     Bypass", "                 Hot Reactor", "                  Separator"] ("BAY 3")
                        w217 = u16 0 items=["                     Bypass", "                Hot Reactor", "                  Separator"] ("BAY 2")
                        w218 = u16 0 items=["                 Bypass", "             Hot Reactor", "               Separator"] ("BAY 1")
                        n201 = local write "BAY 3"(w216) -> ()
                        n202 = local write "BAY 4"(w215) -> ()
                        n203 = local write "BAY 5"(w214) -> ()
                        n204 = local write "BAY 2"(w217) -> ()
                        n205 = local write "BAY 1"(w218) -> ()
                        n206 = local write "Synthesis Route Array"(string[][] [["3-Br-Pyridine _ Biphenyl", "K2CO3", "PhB(OH)2", "", "", ""]] ("Synthesis Route Array")) -> ()
                      }
                    }
                  }
                }
              }
              frame Enabled {
              }
            }
            n207 = disable-structure shown="Disabled" {
              disable-tunnel: 400 -> [w204 _]
              frame Disabled {
                n208 = event shown="[1]" {
                  selector: _ -> [_ _]
                  dyn-events: _ -> [_ _]
                  timeout: w204 -> [_ _]
                  event Timeout {
                    n209 = event-data() -> ()  [unwired: 1 in, 3 out]
                  }
                  event #1 (no event record) {
                    n210 = event-data() -> ()  [unwired: 1 in, 6 out]
                    n211 = call "File Dialog"("prompt"="Load previously saved xml file") -> ("selected path"=w206:path)  [unwired: 11 in, 3 out]
                    n212 = Path To String(path=w206) -> (string=w205:string)
                    n213 = script code="xmlDoc = xmlread(file_path);\nroot = xmlDoc.getDocumentElement();\nb = root.getChildNodes;\nrecipe = b.getElementsByTagName('Bay1').item(0);"("file_path"=w205) -> ()  [unwired: 1 in, 1 out]
                  }
                }
              }
              frame Enabled {
              }
            }
          }
        }
        frame #1 {
          n214 = local read "Stop"() -> (w424:bool)
          n215 = Not(x=w424) -> (.not. x?=w423:bool)
          n216 = case shown="True" w423 {
            tunnel: w425 -> [_ w428]
            frame False {
              "stop_button clicked" <- TRUE ("stop_button clicked")
            }
            frame True {
              # "Parameters Initilization"
              n217 = flat-sequence {
                tunnel: w428 -> [w430]
                tunnel: [w429] -> w427
                tunnel: w427 -> [w589]
                frame #0 {
                  # "Setup bays(RFID - verify)"
                  n218 = disable-structure shown="Disabled" {
                    frame Disabled {
                      n219 = local read "BAY 1"() -> ()  [unwired: 1 out]
                      n220 = local read "BAY 2"() -> ()  [unwired: 1 out]
                      n221 = local read "BAY 3"() -> ()  [unwired: 1 out]
                      n222 = local read "BAY 4"() -> ()  [unwired: 1 out]
                      n223 = local read "BAY 5"() -> ()  [unwired: 1 out]
                    }
                    frame Enabled {
                    }
                  }
                }
                frame #1 {
                  n224 = while {
                    tunnel: w430 -> [w433]
                    tunnel: [w432] -> w429
                    stop <- w436 stop-if-true
                    n225 = flat-sequence {
                      tunnel: [w450] -> w432
                      tunnel: w433 -> [w531]
                      tunnel: [w449] -> w431
                      frame #0 {
                        n226 = while {
                          stop <- w440 stop-if-true
                          n227 = event shown="[1] \"System Parameters Confirm Button\": Value Change" {
                            selector: _ -> [_ _]
                            dyn-events: _ -> [_ _]
                            timeout: u32 200 ("milliseconds to wait") -> [_ _]
                            tunnel: [FALSE TRUE] -> w438
                            event Timeout {
                              n228 = event-data() -> ()  [unwired: 1 in, 3 out]
                            }
                            event "System Parameters Confirm Button": Value Change {
                              n229 = event-data() -> ()  [unwired: 1 in, 5 out]
                              n230 = local write "System Parameters Confirm Button"(FALSE) -> ()
                            }
                          }
                          n231 = Wait (ms)(milliseconds to wait=u32 500) -> ()  [unwired: 1 out]
                          n232 = local read "Stop"() -> (w441:bool)
                          n233 = Or(x=w441, y=w438) -> (x .or. y?=w440:bool)
                        }
                      }
                      frame #1 {
                        w470 = 0 ("disabled index (col)")
                        w482 = 1 ("disabled index (col)")
                        # "Do while parameters have not been correctly entered"
                        n234 = local read "Bay Parameters"() -> (w469:T2)
                        n235 = local read "Synthesis Route Array"() -> (w483:string[][])
                        n236 = local read "Total Number of Experiments"() -> (w502:dbl)
                        n237 = Unbundle By Name(w469) -> ("Continue from previous optimization?"=w530:bool)
                        n238 = Unbundle By Name(w469) -> ("Excel File Name"=w532:string)
                        n239 = Unbundle By Name(w469) -> ("Matlab File"=w528:string)
                        n240 = Unbundle By Name(w469) -> ("Bay 1.Run at set flowrate"=w574:bool)
                        n241 = Unbundle By Name(w469) -> ("Bay 1.Pump 1 Flowrate"=w580:dbl)
                        n242 = Unbundle By Name(w469) -> ("Bay 1.Pump 2 Flowrate"=w579:dbl)
                        n243 = Unbundle By Name(w469) -> ("Bay 2.Run at set flowrate"=w572:bool)
                        n244 = Unbundle By Name(w469) -> ("Bay 2.Pump 3 Flowrate"=w578:dbl)
                        n245 = Unbundle By Name(w469) -> ("Bay 3.Pump 4 Flowrate"=w577:dbl)
                        n246 = Unbundle By Name(w469) -> ("Bay 3.Run at set flowrate"=w571:bool)
                        n247 = Unbundle By Name(w469) -> ("Bay 4.Run at set flowrate"=w568:bool)
                        n248 = Unbundle By Name(w469) -> ("Bay 4.Pump 5 Flowrate"=w576:dbl)
                        n249 = Unbundle By Name(w469) -> ("Bay 5.Pump 6 Flowrate"=w575:dbl)
                        n250 = Unbundle By Name(w469) -> ("Bay 5.Run at set flowrate"=w567:bool)
                        n251 = Index Array(array=w483, index (row)=3, index (col)=w482) -> (element=w476:string)
                        n252 = Index Array(array=w483, index (row)=2, index (col)=w482) -> (element=w474:string)
                        n253 = Index Array(array=w483, index (row)=1, index (col)=w482) -> (element=w472:string)
                        n254 = Index Array(array=w483, index (row)=0, index (col)=w482) -> (element=w485:string)
                        n255 = Index Array(array=w483, index (row)=4, index (col)=w482) -> (element=w478:string)
                        n256 = Index Array(array=w483, index (row)=5, index (col)=w482) -> (element=w480:string)
                        n257 = Build Array(w485, w472, w474, w476, w478, w480) -> (w486:string[])
                        n258 = Index Array(array=w483, index (row)=0 ("index"), index (col)=w470) -> (element=w508:string)
                        n259 = for {
                          tunnel: w486 -> [w582] mode=indexing
                          tunnel: [w581] -> w471 mode=indexing
                          n260 = script code="ctemp1 = str2num(c_temp);"("c_temp"=w582) -> ("ctemp1"=w581:dbl)  [unwired: 1 in, 1 out]
                        }
                        n261 = Boolean To (0,1)(Boolean=w572) -> (0, 1=w527:i16)
                        n262 = Boolean To (0,1)(Boolean=w568) -> (0, 1=w569:i16)
                        n263 = Boolean To (0,1)(Boolean=w571) -> (0, 1=w570:i16)
                        n264 = Boolean To (0,1)(Boolean=w530) -> (0, 1=w529:i16)
                        n265 = Boolean To (0,1)(Boolean=w574) -> (0, 1=w573:i16)
                        n266 = Boolean To (0,1)(Boolean=w567) -> (0, 1=w566:i16)
                        n267 = Index Array(array=w483, index (row)=1 ("index"), index (col)=w470) -> (element=w503:string)
                        n268 = Index Array(array=w483, index (row)=2 ("index"), index (col)=w470) -> (element=w504:string)
                        n269 = Unbundle By Name(w469) -> ("Bay 1.optimize_temp"=w565:bool)
                        n270 = Unbundle By Name(w469) -> ("Bay 1.optimize_tau"=w563:bool)
                        n271 = Unbundle By Name(w469) -> ("Bay 2.optimize_temp"=w561:bool)
                        n272 = Unbundle By Name(w469) -> ("Bay 2.optimize_tau"=w559:bool)
                        n273 = Unbundle By Name(w469) -> ("Bay 3.optimize_temp"=w557:bool)
                        n274 = Unbundle By Name(w469) -> ("Bay 3.optimize_tau"=w555:bool)
                        n275 = Unbundle By Name(w469) -> ("Bay 4.optimize_temp"=w553:bool)
                        n276 = Unbundle By Name(w469) -> ("Bay 4.optimize_tau"=w551:bool)
                        n277 = Index Array(array=w483, index (row)=3 ("index"), index (col)=w470) -> (element=w505:string)
                        n278 = Boolean To (0,1)(Boolean=w553) -> (0, 1=w552:i16)
                        n279 = Boolean To (0,1)(Boolean=w551) -> (0, 1=w550:i16)
                        n280 = Index Array(array=w483, index (row)=4 ("index"), index (col)=w470) -> (element=w506:string)
                        n281 = Boolean To (0,1)(Boolean=w555) -> (0, 1=w554:i16)
                        n282 = Boolean To (0,1)(Boolean=w561) -> (0, 1=w560:i16)
                        n283 = Boolean To (0,1)(Boolean=w565) -> (0, 1=w564:i16)
                        n284 = Boolean To (0,1)(Boolean=w559) -> (0, 1=w558:i16)
                        n285 = Boolean To (0,1)(Boolean=w563) -> (0, 1=w562:i16)
                        n286 = Boolean To (0,1)(Boolean=w557) -> (0, 1=w556:i16)
                        n287 = Unbundle By Name(w469) -> ("Bay 5.optimize_temp"=w549:bool)
                        n288 = Unbundle By Name(w469) -> ("Bay 5.optimize_tau"=w547:bool)
                        n289 = Index Array(array=w483, index (row)=5 ("index"), index (col)=w470) -> (element=w507:string)
                        n290 = Boolean To (0,1)(Boolean=w549) -> (0, 1=w548:i16)
                        n291 = Boolean To (0,1)(Boolean=w547) -> (0, 1=w546:i16)
                        n292 = Build Array(w564, w562, w560, w558, w556, w554, w552, w550, w548, w546) -> (w545:i16[])
                        n293 = Unbundle By Name(w469) -> ("Bay 1.Temperature Params"=w542:dbl[])
                        n294 = Unbundle By Name(w469) -> ("Bay 2.Temperature Params"=w541:dbl[])
                        n295 = Unbundle By Name(w469) -> ("Bay 2.Resisdence time params"=w536:dbl[])
                        n296 = Unbundle By Name(w469) -> ("Bay 3.Temperature Params"=w540:dbl[])
                        n297 = Unbundle By Name(w469) -> ("Bay 3.Resisdence time params"=w535:dbl[])
                        n298 = Unbundle By Name(w469) -> ("Bay 4.Temperature Params"=w539:dbl[])
                        n299 = Unbundle By Name(w469) -> ("Bay 4.Resisdence time params"=w534:dbl[])
                        n300 = Unbundle By Name(w469) -> ("Bay 5.Temperature Params"=w538:dbl[])
                        n301 = Unbundle By Name(w469) -> ("Bay 5.Resisdence time params"=w533:dbl[])
                        n302 = Unbundle By Name(w469) -> ("Bay 1.pump params 2"=w501:dbl[])
                        n303 = Unbundle By Name(w469) -> ("Bay 1.pump params 1"=w537:dbl[])
                        n304 = Unbundle By Name(w469) -> ("Bay 1.Run at set temperature"=w492:bool)
                        n305 = Unbundle By Name(w469) -> ("Bay 2.Run at set temperature"=w490:bool)
                        n306 = Unbundle By Name(w469) -> ("Bay 3.Run at set temperature"=w489:bool)
                        n307 = Unbundle By Name(w469) -> ("Bay 4.Run at set temperature"=w488:bool)
                        n308 = Unbundle By Name(w469) -> ("Bay 5.Run at set temperature"=w487:bool)
                        n309 = Unbundle By Name(w469) -> ("Bay 3.Temperature"=w498:dbl)
                        n310 = Unbundle By Name(w469) -> ("Bay 1.Temperature"=w500:dbl)
                        n311 = Unbundle By Name(w469) -> ("Bay 2.Temperature"=w499:dbl)
                        n312 = Unbundle By Name(w469) -> ("Bay 4.Temperature"=w497:dbl)
                        n313 = Unbundle By Name(w469) -> ("Bay 5.Temperature"=w496:dbl)
                        n314 = Unbundle By Name(w469) -> ("Bay 3.pump_num_ratio"=w521:dbl)
                        n315 = Unbundle By Name(w469) -> ("Bay 4.pump_num_ratio"=w518:dbl)
                        n316 = Unbundle By Name(w469) -> ("Bay 5.pump_num_ratio"=w515:dbl)
                        n317 = Unbundle By Name(w469) -> ("Bay 2.pump_num_ratio"=w524:dbl)
                        n318 = Unbundle By Name(w469) -> ("Bay 4.pump_at_ratio"=w520:bool)
                        n319 = Boolean To (0,1)(Boolean=w520) -> (0, 1=w519:i16)
                        n320 = Unbundle By Name(w469) -> ("Bay 3.pump_at_ratio"=w523:bool)
                        n321 = Boolean To (0,1)(Boolean=w523) -> (0, 1=w522:i16)
                        n322 = Unbundle By Name(w469) -> ("Bay 5.pump_at_ratio"=w517:bool)
                        n323 = Boolean To (0,1)(Boolean=w517) -> (0, 1=w516:i16)
                        n324 = Unbundle By Name(w469) -> ("Bay 2.pump_at_ratio"=w526:bool)
                        n325 = Boolean To (0,1)(Boolean=w526) -> (0, 1=w525:i16)
                        n326 = Build Array(w500, w499, w498, w497, w496) -> (w495:dbl[])
                        n327 = Build Array(w492, w490, w489, w488, w487) -> (w491:bool[])
                        n328 = local read "Syringe_pump?"() -> (w448:bool)
                        n329 = for {
                          N: 5 -> [_]
                          tunnel: w491 -> [w586] mode=indexing
                          tunnel: [w585] -> w493 mode=indexing
                          n330 = Select(t=1.0, s=w586, f=0.0) -> (s? t:f=w585:dbl)
                        }
                        n331 = Unbundle By Name(w469) -> ("Internal Standard?"=w460:bool)
                        n332 = Unbundle By Name(w469) -> ("increas_decrease_hplc_peak"=w461:bool)
                        n333 = Unbundle By Name(w469) -> ("Hplc Wait time(min)"=w453:dbl)
                        n334 = Unbundle By Name(w469) -> ("Total Number of Experiments 2"=w452:dbl)
                        n335 = Unbundle By Name(w469) -> ("hplc_start"=w457:dbl)
                        n336 = Unbundle By Name(w469) -> ("ISTD start"=w455:dbl)
                        n337 = Unbundle By Name(w469) -> ("hplc_end"=w456:dbl)
                        n338 = Unbundle By Name(w469) -> ("throughput_yield"=w462:bool)
                        n339 = Unbundle By Name(w469) -> ("ISTD end"=w454:dbl)
                        n340 = Select(t=1.0, s=w448, f=0.0) -> (s? t:f=w447:dbl)
                        n341 = Select(t=1.0, s=w461, f=0.0) -> (s? t:f=w459:dbl)
                        n342 = Select(t=1.0, s=w460, f=0.0) -> (s? t:f=w458:dbl)
                        n343 = Select(t=0.0, s=w462, f=1.0) -> (s? t:f=w451:dbl)
                        n344 = script code="system_error = 0;\nnumPeaks = 1;\nstart_phase_time = 1;\nis_redo_exp = 0;\nFvalues = [];\nHPLC_Area = [];\n\nT1_span = [1 1]; T2_span = [1 1]; T3_span = [1 1]; T4_span = [1 1]; T5_span = [1 1];\nT_span = [T1_span;T2_span;T3_span;T4_span;T5_span];\n p1_span =  [1 1]; p2_span =  [1 1]; p3_span =  [1 1]; p4_span =  [1 1]; p5_span =  [1 1];  p6_span =  [1 1];\nOpt_params = [0 0 0 0 0 0 0 0 0 0 0];\nT_params = [T1_params;T2_params;T3_params;T4_params;T5_params];\npump_params = [pump1_params;pump2_params;pump3_params;pump4_params;pump5_params;pump6_params];\nopt_ctr = 0;ncall = 100;record_data = true;\nT1_SP = 23; T2_SP = 23; T3_SP = 23; T4_SP = 23; T5_SP = 23;\nT_span = [T1_span;T2_span;T3_span;T4_span;T5_span];\np_span = [p1_span;p2_span;p3_span;p4_span;p5_span;p6_span];\nno_errors = 1;\nP1 = 0; P2 =0; P3 = 0; P4 = 0; P5 = 0; P6 = 0;\nP = [P1, P2, P3,P4, P5, P6];\nis_first_set_of_exp = true;\nerror_message = 'System has no errors to report';\naddpath(genpath('C:\\Users\\HPLC\\Dropbox (MIT)\\MoD Files\\MATLAB'))\n%addpath(genpath('C:\\Users\\Admin\\Dropbox (MIT)\\MoD Files\\MATLAB'))\nallMSData = [];allHPLCData = [];allHPLCFile = [];\nBay_ratio = [0,Bay2_ratio,Bay3_ratio,Bay4_ratio,Bay5_ratio];\nBay_pump_ratio = [1, Bay2_pump_ratio, Bay3_pump_ratio, Bay4_pump_ratio, Bay5_pump_ratio];\nP_setrate = [P1_setrate, P2_setrate, P3_setrate, P4_setrate, P5_setrate, P6_setrate];\nuse_flowrate = [use_flowrate1, use_flowrate2,use_flowrate3, use_flowrate4, use_flowrate5];\npump_chem_name= []\nCurrExp = 1;\n% ****************************************************************************************************\n%Setup optimization\n   setup_optimization_params;\n   initialize_opt = 0;\n   nstop0 = 0;\n%*****************************************************************************************************\n% Setup excel and xml file writing\npath(path, pa);\nnumMSSig = 1;\nsetup_excel_output;\n%***************************************************************************************************\nredo = false;\nncall = ncall_in;"("use_flowrate1"=w573, "P1_setrate"=w580, "P2_setrate"=w579, "P3_setrate"=w578, "P4_setrate"=w577, "P5_setrate"=w576, "P6_setrate"=w575, "use_flowrate2"=w527, "use_flowrate3"=w570, "use_flowrate4"=w569, "use_flowrate5"=w566, "Optimize_params"=w545, "T1_params"=w542, "T2_params"=w541, "T3_params"=w540, "T4_params"=w539, "T5_params"=w538, "pump1_params"=w537, "pump3_params"=w536, "pump4_params"=w535, "pump5_params"=w534, "pump6_params"=w533, "xl_file"=w532, "pa"=w531, "Continue"=w529, "matlabsavefile"=w528, "Bay2_ratio"=w525, "Bay2_pump_ratio"=w524, "Bay3_ratio"=w522, "Bay3_pump_ratio"=w521, "Bay4_ratio"=w519, "Bay4_pump_ratio"=w518, "Bay5_ratio"=w516, "Bay5_pump_ratio"=w515, "pump1_chem"=w508, "pump6_chem"=w507, "pump5_chem"=w506, "pump4_chem"=w505, "pump3_chem"=w504, "pump2_chem"=w503, "Pump_concen"=w471, "ncall_in"=w502, "pump2_params"=w501, "T_SP"=w495, "Run_at_T_SP"=w493, "dcr_hplc_peak"=w459, "use_internal_std"=w458, "hplc_peak_start"=w457, "hplc_peak_end"=w456, "ISTD_start"=w455, "ISTD_end"=w454, "hplc_wait_time"=w453, "tot_num_exp"=w452, "throughput_yield"=w451, "syringe_pump"=w447) -> ("no_errors"=w544:dbl, "error_message"=w543:string)  [unwired: 1 in, 1 out]
                        n345 = Not Equal To 0?(x=w544) -> (x != 0?=w449:bool)
                        n346 = Not(x=w449) -> (.not. x?=w450:bool)
                        n347 = case shown="False" w450 {
                          tunnel: w543 -> [_ w588]
                          frame False {
                            n348 = local write "Setup Confirm 2"(TRUE ("Setup Confirm 2")) -> ()
                          }
                          frame True {
                            n349 = One Button Dialog(message=w588) -> ()  [unwired: 1 in, 1 out]
                          }
                        }
                      }
                    }
                    n350 = local read "Stop"() -> (w435:bool)
                    n351 = Or(x=w431, y=w435) -> (x .or. y?=w436:bool)
                    n352 = Wait (ms)(milliseconds to wait=u32 500) -> ()  [unwired: 1 out]
                  }
                }
                frame #2 {
                  n353 = local write "System Error"(w589) -> ()
                }
              }
            }
          }
        }
        frame #2 {
          # "Run Initial diagnostics"
        }
        frame #3 {
          # "Run System"
          n354 = while {
            tunnel: w590 -> [w1263]
            stop <- w1267 stop-if-true
            n355 = local read "running?"() -> (w1262:bool)
            n356 = local read "Temperature Control 1"() -> (w1264:bool)
            n357 = And(x=w1262, y=w1264) -> (x .and. y?=w1265:bool)
            n358 = case shown="True" w1265 {
              tunnel: w1263 -> [_ w1269]
              frame False {
                n359 = local write "Temp SS? 1"(TRUE ("Temp SS? 1")) -> ()
              }
              frame True {
                # "Bay 1 Temperature Controller"
                n360 = local read "Temperature SP 1"() -> (w1270:dbl)
                n361 = local read "Temperature 1"() -> (w1274:dbl)
                n362 = local read "SSR Duration 1"() -> (w1289:dbl)
                n363 = call-poly <vilib>:"PID Online Autotuning.vi"("setpoint"=w1270, "manipulated variable"=w1289, "autotuning parameters"=T9 {"type of controller"=enum."PID", "relay cycles"=3, "relay amplitude"=1.0, "control specifications"=enum."Normal", "PV noise level"=0.1} ("Autotuning Parameters R1"), "process variable"=w1274, "PID gains in"=T8 {"Proportional gain Kc"=0.38538, "Integral time Ti (sec)"=0.524375, "Derivative time Ti (sec)"=0.12585} ("PID gains 2")) -> ("setpoint out"=w1295:dbl, "process variable out"=w1294:dbl, "PID gains out"=w1291:T17)  [unwired: 6 in, 2 out]
                n364 = call <vilib>:"PID Autotuning (Temperature).vi"("desired temperature"=w1295, "measured temperature"=w1294, "plant parameters in"=w1291, "output range"=cluster{"output high":dbl, "output low":dbl} {"output high"=3.0, "output low"=-1.0} ("Output range")) -> ("output"=w1287:dbl)  [unwired: 12 in, 3 out]
                n365 = local write "SSR Duration 1"(w1287) -> ()
                n366 = Subtract(x=w1270, y=w1274) -> (x-y=w1281:dbl)
                n367 = Absolute Value(x=w1281) -> (abs(x)=w1284:dbl)
                n368 = Multiply(x=1000.0, y=w1287) -> (x*y=w1285:dbl)
                n369 = Greater Than 0?(x=w1285) -> (x > 0?=w1279:bool)
                n370 = Less Or Equal?(x=w1284, y=1.2) -> (x <= y?=w1282:bool)
                n371 = Greater?(x=w1270, y=w1274) -> (0:w1280:bool)
                n372 = And(x=w1279, y=w1280) -> (x .and. y?=w1277:bool)
                n373 = local write "Temp SS? 1"(w1282) -> ()
                n374 = Subtract(x=w1274, y=10.0) -> (x-y=w1275:dbl)
                n375 = Less?(x=w1275, y=w1270) -> (x < y?=w1278:bool)
                n376 = And(x=w1278, y=w1277) -> (x .and. y?=w1276:bool)
                n377 = case shown="True" w1276 {
                  tunnel: [errorcluster {"status"=FALSE, "code"=0, "source"=""} ("error out") w1305] -> _
                  tunnel: 2 -> [_ w1302]
                  tunnel: w1285 -> [w1299 w1303]
                  tunnel: [0.0 w1307] -> w1272
                  tunnel: w1270 -> [_ w1306]
                  tunnel: w1269 -> [_ w1304]
                  frame False {
                    n378 = Absolute Value(x=w1299) -> (abs(x)=w1300:dbl)
                    n379 = Wait (ms)(milliseconds to wait=w1300) -> ()  [unwired: 1 out]
                  }
                  frame True {
                    n380 = call "TurnOnRelayArduino.vi"("channel"=w1302, "duration"=w1303, "LINX Resource"=w1304) -> ("error out"=w1305:errorcluster)  [unwired: 7 in, 1 out]
                    n381 = script code="tempdiff1= SP1 - T1;\nif tempdiff1 > 10\n  if slope1 < .01\n     temp_check1 = temp_check1 + 1;\n  else\n      temp_check1 =0;\n  end\nend\n\nif temp_check1 > 9\n  temp_error1 = 1\nend"("SP1"=w1306) -> ("temp_error1"=w1307:dbl)  [unwired: 1 in, 1 out]
                  }
                }
                n382 = Not Equal To 0?(x=w1272) -> (x != 0?=w1271:bool)
                n383 = case shown="True" w1271 {
                  frame False {
                  }
                  frame True {
                    n384 = local write "Error Message"("Bay 1 Temperature Heating Error") -> ()
                  }
                }
                n385 = case shown="True" w1271 {
                  tunnel: w1271 -> [_ w1297]
                  frame False {
                  }
                  frame True {
                    n386 = local write "System Error"(w1297) -> ()
                    n387 = local write "Stop"(w1297) -> ()
                  }
                }
              }
            }
            n388 = Wait (ms)(milliseconds to wait=u32 400) -> ()  [unwired: 1 out]
            n389 = local read "Stop"() -> (w1267:bool)
          }
          n390 = local read "Bay Parameters"() -> (w594:T2)
          n391 = while {
            tunnel: w590 -> [w1217]
            stop <- w1221 stop-if-true
            n392 = local read "running?"() -> (w1216:bool)
            n393 = local read "Temperature Control 2"() -> (w1218:bool)
            n394 = And(x=w1216, y=w1218) -> (x .and. y?=w1219:bool)
            n395 = case shown="True" w1219 {
              tunnel: w1217 -> [_ w1223]
              frame False {
                n396 = local write "Temp SS? 2"(TRUE ("Temp SS? 2")) -> ()
              }
              frame True {
                # "Bay 2 Temperature Controller"
                n397 = local read "Temperature SP 2"() -> (w1225:dbl)
                n398 = local read "Temperature 2"() -> (w1228:dbl)
                n399 = local read "SSR Duration 2"() -> (w1246:dbl)
                n400 = call-poly <vilib>:"PID Online Autotuning.vi"("setpoint"=w1225, "manipulated variable"=w1246, "autotuning parameters"=T9 {"type of controller"=enum."PID", "relay cycles"=3, "relay amplitude"=1.0, "control specifications"=enum."Normal", "PV noise level"=0.1} ("Autotuning Parameters R1"), "process variable"=w1228, "PID gains in"=T8 {"Proportional gain Kc"=0.38538, "Integral time Ti (sec)"=0.524375, "Derivative time Ti (sec)"=0.12585} ("PID gains 2")) -> ("setpoint out"=w1244:dbl, "process variable out"=w1243:dbl, "PID gains out"=w1249:T17)  [unwired: 6 in, 2 out]
                n401 = call <vilib>:"PID Autotuning (Temperature).vi"("desired temperature"=w1244, "measured temperature"=w1243, "plant parameters in"=w1249, "output range"=cluster{"output high":dbl, "output low":dbl} {"output high"=3.0, "output low"=-1.0} ("Output range")) -> ("output"=w1239:dbl)  [unwired: 12 in, 3 out]
                n402 = local write "SSR Duration 2"(w1239) -> ()
                n403 = Greater?(x=w1225, y=w1228) -> (0:w1234:bool)
                n404 = Multiply(x=1000.0, y=w1239) -> (x*y=w1241:dbl)
                n405 = Greater Than 0?(x=w1241) -> (x > 0?=w1233:bool)
                n406 = And(x=w1233, y=w1234) -> (x .and. y?=w1231:bool)
                n407 = Subtract(x=w1225, y=w1228) -> (x-y=w1236:dbl)
                n408 = Absolute Value(x=w1236) -> (abs(x)=w1238:dbl)
                n409 = Subtract(x=w1228, y=10.0) -> (x-y=w1230:dbl)
                n410 = Less Or Equal?(x=w1238, y=1.2) -> (x <= y?=w1235:bool)
                n411 = local write "Temp SS? 2"(w1235) -> ()
                n412 = Less?(x=w1230, y=w1225) -> (x < y?=w1232:bool)
                n413 = And(x=w1232, y=w1231) -> (x .and. y?=w1227:bool)
                n414 = case shown="True" w1227 {
                  tunnel: [errorcluster {"status"=FALSE, "code"=0, "source"=""} ("error out") w1259] -> _
                  tunnel: 3 -> [_ w1256]
                  tunnel: w1241 -> [w1253 w1257]
                  tunnel: [0.0 w1261] -> w1226
                  tunnel: w1225 -> [_ w1260]
                  tunnel: w1223 -> [_ w1258]
                  frame False {
                    n415 = Absolute Value(x=w1253) -> (abs(x)=w1254:dbl)
                    n416 = Wait (ms)(milliseconds to wait=w1254) -> ()  [unwired: 1 out]
                  }
                  frame True {
                    n417 = call "TurnOnRelayArduino.vi"("channel"=w1256, "duration"=w1257, "LINX Resource"=w1258) -> ("error out"=w1259:errorcluster)  [unwired: 7 in, 1 out]
                    n418 = script code="tempdiff2= SP2 - T2;\nif tempdiff2 > 10\n  if slope2 < .01\n     temp_check2 = temp_check2 + 1;\n  else\n      temp_check2 =0;\n  end\nend\n\nif temp_check2 > 9\n  temp_error2 = 1\nend"("SP2"=w1260) -> ("temp_error2"=w1261:dbl)  [unwired: 1 in, 1 out]
                  }
                }
                n419 = Not Equal To 0?(x=w1226) -> (x != 0?=w1224:bool)
                n420 = case shown="True" w1224 {
                  frame False {
                  }
                  frame True {
                    n421 = local write "Error Message"("Bay 2 Temperature Heating Error") -> ()
                  }
                }
                n422 = case shown="True" w1224 {
                  tunnel: w1224 -> [_ w1251]
                  frame False {
                  }
                  frame True {
                    n423 = local write "Stop"(w1251) -> ()
                    n424 = local write "System Error"(w1251) -> ()
                  }
                }
              }
            }
            n425 = local read "Stop"() -> (w1221:bool)
            n426 = Wait (ms)(milliseconds to wait=u32 400) -> ()  [unwired: 1 out]
          }
          n427 = local read "Stop"() -> (w591:bool)
          n428 = Not(x=w591) -> (.not. x?=w593:bool)
          n429 = case shown="True" w593 {
            tunnel: w594 -> [_ w599]
            tunnel: w592 -> [_ w598]
            tunnel: w590 -> [_ w597]
            frame False {
            }
            frame True {
              n430 = while {
                tunnel: w599 -> [w613]
                tunnel: w598 -> [w605]
                tunnel: w597 -> [w600]
                i -> [w612]
                stop <- w606 stop-if-true
                n431 = local read "running?"() -> (w601:bool)
                n432 = Wait (ms)(milliseconds to wait=u32 1000) -> ()  [unwired: 1 out]
                n433 = Increment(x=w612) -> (x+1=w602:i32)
                n434 = case shown="True" w601 {
                  tunnel: w612 -> [w618 _]
                  tunnel: w613 -> [_ _]
                  tunnel: [w620 w624] -> w603
                  tunnel: [0.0 w625] -> w608
                  tunnel: w605 -> [_ w623]
                  tunnel: w600 -> [_ w621]
                  frame False {
                    # "STANDBY MODE"
                    n435 = Add(x=w618, y=2.0) -> (x+y=w620:dbl)
                  }
                  frame True {
                    n436 = flat-sequence {
                      tunnel: w623 -> [w627]
                      tunnel: [w627] -> w622
                      tunnel: [w639] -> w625
                      tunnel: [200.0] -> w624
                      tunnel: w622 -> [w637]
                      tunnel: w621 -> [w628]
                      frame #0 {
                        n437 = local write "stop_xl_write"(FALSE ("stop_xl_write")) -> ()
                      }
                      frame #1 {
                        # "Increase flowrate of dilution stream"
                        # "Wait mixed stream reaches SL"
                        # "SNOBFIT"
                        # "Optimize"
                        # "Run Experimental Conditions"
                        # "Optimize/Synthesize"
                        n438 = local read "Syringe_pump?"() -> (w631:bool)
                        n439 = local read "Stop"() -> (w634:bool)
                        n440 = Not(x=w634) -> (.not. x?=w633:bool)
                        n441 = case shown="True" w633 {
                          tunnel: [1.0 w661] -> w642
                          tunnel: [w649 w660] -> w636
                          tunnel: [0.0 w659] -> w635
                          tunnel: [w649 w658] -> w632
                          tunnel: w631 -> [_ w655]
                          frame False {
                            w649 = dbl[] []
                          }
                          frame True {
                            n442 = Select(t=1.0, s=w655, f=0.0) -> (s? t:f=w654:dbl)
                            n443 = script code="optimization_main_loop"("syringe_pump"=w654) -> ("Conditions_Array"=w660:dbl[], "opt_ctr"=w661:dbl, "P_tot"=w659:dbl, "tau_array"=w658:dbl[], "experiment_history"=w656:dbl[][])  [unwired: 1 in, 1 out]
                            n444 = call-poly <vilib>:"Array To Matrix.vi"("Real 2D Array"=w656) -> ("Real Matrix"=w657:T18)
                            n445 = local write "experiment history"(w657) -> ()
                          }
                        }
                        "P_tot" <- w635
                        n446 = local read "COMM Port :: Milligat Pumps"() -> (w643:refnum<visa-resource-name>)
                        n447 = Equal?(x=w642, y=1.0) -> (x = y?=w640:bool)
                        n448 = flat-sequence {
                          tunnel: w636 -> [w1061]
                          tunnel: w632 -> [w1055]
                          frame #0 {
                            # "Start recording data"
                            n449 = Index Array(array=w1061, index=5) -> (element=w1073:dbl)
                            n450 = Index Array(array=w1061, index=0) -> (element=w1068:dbl)
                            n451 = Index Array(array=w1061, index=1) -> (element=w1069:dbl)
                            n452 = Index Array(array=w1061, index=2) -> (element=w1071:dbl)
                            n453 = Index Array(array=w1061, index=3) -> (element=w1070:dbl)
                            n454 = Index Array(array=w1061, index=4) -> (element=w1072:dbl)
                            n455 = local write "Pump setpoint(ul/min) 2"(w1069) -> ()
                            n456 = local write "Pump setpoint(ul/min) 3"(w1071) -> ()
                            n457 = local write "Pump setpoint(ul/min) 5"(w1072) -> ()
                            n458 = local write "Pump setpoint(ul/min) 4"(w1070) -> ()
                            n459 = local write "Pump setpoint(ul/min) 6"(w1073) -> ()
                            n460 = local write "Pump setpoint(ul/min) 1"(w1068) -> ()
                            n461 = Index Array(array=w1055, index=0) -> (element=w1060:dbl)
                            n462 = Index Array(array=w1055, index=4) -> (element=w1059:dbl)
                            n463 = Index Array(array=w1055, index=3) -> (element=w1058:dbl)
                            n464 = Index Array(array=w1055, index=2) -> (element=w1057:dbl)
                            n465 = Index Array(array=w1055, index=1) -> (element=w1056:dbl)
                            n466 = local write "tau 2"(w1056) -> ()
                            n467 = local write "tau 3"(w1057) -> ()
                            n468 = local write "tau 4"(w1058) -> ()
                            n469 = local write "tau 5"(w1059) -> ()
                            n470 = local write "tau 1"(w1060) -> ()
                          }
                        }
                        n471 = flat-sequence {
                          tunnel: w643 -> [w665]
                          tunnel: w636 -> [w664]
                          tunnel: w640 -> [w663]
                          tunnel: [w663] -> w648
                          tunnel: w637 -> [w662]
                          tunnel: w648 -> [w819]
                          tunnel: [w819] -> w647
                          tunnel: w647 -> [w839]
                          tunnel: [w837] -> w630
                          tunnel: w630 -> [w861]
                          tunnel: [w861] -> w629
                          tunnel: w628 -> [_]
                          tunnel: w636 -> [w864]
                          tunnel: w629 -> [w863]
                          tunnel: w628 -> [w862]
                          tunnel: [w991] -> w646
                          tunnel: w646 -> [w1004]
                          tunnel: [w1004] -> w645
                          tunnel: w645 -> [w1012]
                          tunnel: [w1012] -> w644
                          tunnel: [w1049] -> w639
                          tunnel: w644 -> [w1049]
                          frame #0 {
                            # "Setup pump flowrates and temperature setpoints"
                            n472 = stacked-sequence {
                              tunnel: w665 -> [w688 _ _ _ _]
                              tunnel: w665 -> [_ w731 _ _ _]
                              tunnel: w665 -> [_ _ w759 _ _]
                              tunnel: w665 -> [_ _ _ w784 _]
                              tunnel: w665 -> [_ _ _ _ w809]
                              tunnel: w664 -> [w685 w729 w757 w782 w806]
                              tunnel: w663 -> [w675 w722 w752 w775 w800]
                              tunnel: w662 -> [w673 _ _ _ _]
                              frame #0 {
                                # "Bay 1"
                                n473 = local read "Syringe_pump?"() -> (w674:bool)
                                n474 = Index Array(array=w685, index=0) -> (element=w683:dbl)
                                n475 = local read "BAY 1"() -> (w668:u16)
                                n476 = Index Array(array=w685, index=1) -> (element=w682:dbl)
                                n477 = Index Array(array=w685, index=6) -> (element=w681:dbl)
                                n478 = script code="MATLAB script"("T1_SP"=w681) -> ()  [unwired: 1 in, 1 out]
                                n479 = Less Or Equal?(x=w668, y=u16 4) -> (x <= y?=w670:bool)
                                n480 = Greater Or Equal?(x=w668, y=u16 1) -> (x >= y?=w671:bool)
                                n481 = And(x=w671, y=w670) -> (x .and. y?=w672:bool)
                                n482 = Greater Than 0?(x=w683) -> (x > 0?=w680:bool)
                                n483 = And(x=w680, y=w675) -> (x .and. y?=w679:bool)
                                n484 = Greater Than 0?(x=w682) -> (x > 0?=w678:bool)
                                n485 = Wait (ms)(milliseconds to wait=u32 300) -> ()  [unwired: 1 out]
                                n486 = And(x=w678, y=w675) -> (x .and. y?=w677:bool)
                                n487 = And(x=w672, y=w675) -> (x .and. y?=w676:bool)
                                n488 = case shown="False" w674 {
                                tunnel: w688 -> [w691 _]
                                tunnel: w682 -> [w690 w698]
                                tunnel: w677 -> [w689 w699]
                                tunnel: w673 -> [_ w697]
                                frame False {
                                n489 = case shown="True" w689 {
                                tunnel: w691 -> [w693 w695]
                                tunnel: w690 -> [_ w694]
                                frame False {
                                n490 = call "PumpStop.vi"("Pump Address"="g", "Pump COMM Port"=w693) -> ()  [unwired: 9 in, 1 out]
                                }
                                frame True {
                                n491 = call "PumpDispense.vi"("Flowrate(ul/min)"=w694, "Pump Address"="g", "Pump COMM Port"=w695) -> ()  [unwired: 7 in, 2 out]
                                }
                                }
                                }
                                frame True {
                                n492 = case shown="True" w699 {
                                tunnel: w698 -> [_ w701]
                                tunnel: w697 -> [w700 w702]
                                frame False {
                                n493 = call <instrlib>:"Stop Pump.vi"("VISA resource name"=w700) -> ()  [unwired: 9 in, 2 out]
                                }
                                frame True {
                                w703 = u16 0 items=["Infuse", "Withdraw"] ("Run Direction (0:Infuse)")
                                w704 = u32 4 items=["milliliters per hour (ml/hr)", "milliliters per minute (ml/min)", "milliliters per second (ml/sec)", "microliters per hour (ul/hr)", "microliters per minute (ul/min)", "microliters per second (ul/sec)", "nanoliters per hour (nl/hr)", "nanoliters per minute (nl/min)", "nanoliters per second (nl/sec)", "picoliters per hour (pl/hr)", "picoliters per minute (pl/min)", "picoliters per second (pl/sec)"] ("Flow Rate Units (1:ml/min)")
                                w705 = u16 0 items=["Infuse", "Withdraw"] ("Pump Direction (0:Infuse)")
                                n494 = call <instrlib>:"Configure Flow Rate & Direction.vi"("VISA resource name"=w702, "Pump Direction (0:Infuse)"=w705, "Flow Rate (5.00)"=w701, "Flow Rate Units (1:ml/min)"=w704) -> ("VISA resource name out"=w706:refnum<visa-resource-name>)  [unwired: 10 in, 1 out]
                                n495 = call <instrlib>:"Start Pump.vi"("Run Direction (0:Infuse)"=w703, "VISA resource name"=w706) -> ()  [unwired: 8 in, 2 out]
                                }
                                }
                                }
                                }
                                n496 = case shown="False" w679 {
                                tunnel: w688 -> [w710 w712]
                                tunnel: w683 -> [_ w713]
                                frame False {
                                n497 = call "PumpStop.vi"("Pump Address"="j", "Pump COMM Port"=w710) -> ()  [unwired: 9 in, 1 out]
                                }
                                frame True {
                                n498 = call "PumpDispense.vi"("Flowrate(ul/min)"=w713, "Pump Address"="j", "Pump COMM Port"=w712) -> ()  [unwired: 7 in, 2 out]
                                }
                                }
                                n499 = case shown="True" w676 {
                                tunnel: w681 -> [_ w709]
                                frame False {
                                n500 = local write "Temperature Control 1"(FALSE) -> ()
                                }
                                frame True {
                                n501 = local write "Temperature SP 1"(w709) -> ()
                                n502 = local write "Temperature Control 1"(TRUE ("Temperature Control 1")) -> ()
                                }
                                }
                              }
                              frame #1 {
                                # "Bay 2"
                                n503 = local read "BAY 2"() -> (w718:u16)
                                n504 = Index Array(array=w729, index=2) -> (element=w726:dbl)
                                n505 = Index Array(array=w729, index=7) -> (element=w727:dbl)
                                n506 = script code="MATLAB script"("T2_SP"=w727) -> ()  [unwired: 1 in, 1 out]
                                n507 = Greater Than 0?(x=w726) -> (x > 0?=w724:bool)
                                n508 = And(x=w724, y=w722) -> (x .and. y?=w723:bool)
                                n509 = Greater Or Equal?(x=w718, y=u16 1) -> (x >= y?=w716:bool)
                                n510 = Less Or Equal?(x=w718, y=u16 4) -> (x <= y?=w721:bool)
                                n511 = And(x=w716, y=w721) -> (x .and. y?=w720:bool)
                                n512 = And(x=w720, y=w722) -> (x .and. y?=w725:bool)
                                n513 = case shown="True" w725 {
                                tunnel: w727 -> [_ w738]
                                frame False {
                                n514 = local write "Temperature Control 2"(FALSE) -> ()
                                }
                                frame True {
                                n515 = local write "Temperature Control 2"(TRUE ("Temperature Control 2")) -> ()
                                n516 = local write "Temperature SP 2"(w738) -> ()
                                }
                                }
                                n517 = case shown="False" w723 {
                                tunnel: w726 -> [_ w734]
                                tunnel: w731 -> [w732 w735]
                                frame False {
                                n518 = call "PumpStop.vi"("Pump Address"="i", "Pump COMM Port"=w732) -> ()  [unwired: 9 in, 1 out]
                                }
                                frame True {
                                n519 = call "PumpDispense.vi"("Flowrate(ul/min)"=w734, "Pump Address"="i", "Pump COMM Port"=w735) -> ()  [unwired: 7 in, 2 out]
                                }
                                }
                                n520 = Wait (ms)(milliseconds to wait=u32 300) -> ()  [unwired: 1 out]
                              }
                              frame #2 {
                                # "Bay 3"
                                n521 = local read "BAY 3"() -> (w747:u16)
                                n522 = Index Array(array=w757, index=3) -> (element=w755:dbl)
                                n523 = Not Equal To 0?(x=w755) -> (x != 0?=w754:bool)
                                n524 = Index Array(array=w757, index=8) -> (element=w742:dbl)
                                n525 = script code="MATLAB script"("T3_SP"=w742) -> ()  [unwired: 1 in, 1 out]
                                n526 = Less Or Equal?(x=w747, y=u16 4) -> (x <= y?=w751:bool)
                                n527 = Greater Or Equal?(x=w747, y=u16 1) -> (x >= y?=w748:bool)
                                n528 = And(x=w748, y=w751) -> (x .and. y?=w746:bool)
                                n529 = And(x=w746, y=w752) -> (x .and. y?=w744:bool)
                                n530 = And(x=w754, y=w752) -> (x .and. y?=w753:bool)
                                n531 = Not Equal?(x=w742, y=23.0) -> (x != y?=w743:bool)
                                n532 = And(x=w744, y=w743) -> (x .and. y?=w740:bool)
                                n533 = case shown="True" w753 {
                                tunnel: w755 -> [_ w762]
                                tunnel: w759 -> [w760 w763]
                                frame False {
                                n534 = call "PumpStop.vi"("Pump Address"="f", "Pump COMM Port"=w760) -> ()  [unwired: 9 in, 1 out]
                                }
                                frame True {
                                n535 = call "PumpDispense.vi"("Flowrate(ul/min)"=w762, "Pump Address"="f", "Pump COMM Port"=w763) -> ()  [unwired: 7 in, 2 out]
                                }
                                }
                                n536 = case shown="True" w740 {
                                tunnel: w742 -> [_ w766]
                                frame False {
                                n537 = local write "Temperature Control 3"(FALSE) -> ()
                                }
                                frame True {
                                n538 = local write "Temperature Control 3"(TRUE ("Temperature Control 3")) -> ()
                                n539 = local write "Temperature SP 3"(w766) -> ()
                                }
                                }
                                n540 = Wait (ms)(milliseconds to wait=u32 300) -> ()  [unwired: 1 out]
                              }
                              frame #3 {
                                # "Bay 4"
                                n541 = Index Array(array=w782, index=9) -> (element=w779:dbl)
                                n542 = script code="MATLAB script"("T4_SP"=w779) -> ()  [unwired: 1 in, 1 out]
                                n543 = Index Array(array=w782, index=4) -> (element=w780:dbl)
                                n544 = Not Equal To 0?(x=w780) -> (x != 0?=w778:bool)
                                n545 = local read "BAY 4"() -> (w769:u16)
                                n546 = And(x=w778, y=w775) -> (x .and. y?=w777:bool)
                                n547 = Less Or Equal?(x=w769, y=u16 4) -> (x <= y?=w774:bool)
                                n548 = Greater Or Equal?(x=w769, y=u16 1) -> (x >= y?=w771:bool)
                                n549 = And(x=w771, y=w774) -> (x .and. y?=w770:bool)
                                n550 = And(x=w770, y=w775) -> (x .and. y?=w776:bool)
                                n551 = case shown="True" w777 {
                                tunnel: w784 -> [w785 w788]
                                tunnel: w780 -> [_ w787]
                                frame False {
                                n552 = call "PumpStop.vi"("Pump Address"="e", "Pump COMM Port"=w785) -> ()  [unwired: 9 in, 1 out]
                                }
                                frame True {
                                n553 = call "PumpDispense.vi"("Flowrate(ul/min)"=w787, "Pump Address"="e", "Pump COMM Port"=w788) -> ()  [unwired: 7 in, 2 out]
                                }
                                }
                                n554 = case shown="True" w776 {
                                tunnel: w779 -> [_ w791]
                                frame False {
                                n555 = local write "Temperature Control 4"(FALSE ("Temperature Control 4")) -> ()
                                }
                                frame True {
                                n556 = local write "Temperature SP 4"(w791) -> ()
                                n557 = local write "Temperature Control 4"(TRUE ("Temperature Control 5")) -> ()
                                }
                                }
                                n558 = Wait (ms)(milliseconds to wait=u32 300) -> ()  [unwired: 1 out]
                              }
                              frame #4 {
                                # "Bay 5"
                                n559 = Index Array(array=w806, index=5) -> (element=w804:dbl)
                                n560 = Index Array(array=w806, index=4) -> (element=w805:dbl)
                                n561 = script code="MATLAB script"("T5_SP"=w805) -> ()  [unwired: 1 in, 1 out]
                                n562 = local read "BAY 5"() -> (w795:u16)
                                n563 = Not Equal To 0?(x=w804) -> (x != 0?=w802:bool)
                                n564 = And(x=w802, y=w800) -> (x .and. y?=w801:bool)
                                n565 = Less Or Equal?(x=w795, y=u16 4) -> (x <= y?=w799:bool)
                                n566 = Greater Or Equal?(x=w795, y=u16 1) -> (x >= y?=w796:bool)
                                n567 = case shown="False" w801 {
                                tunnel: w809 -> [w810 w813]
                                tunnel: w804 -> [_ w812]
                                frame False {
                                n568 = call "PumpStop.vi"("Pump Address"="h", "Pump COMM Port"=w810) -> ()  [unwired: 9 in, 1 out]
                                }
                                frame True {
                                n569 = call "PumpDispense.vi"("Flowrate(ul/min)"=w812, "Pump Address"="h", "Pump COMM Port"=w813) -> ()  [unwired: 7 in, 2 out]
                                }
                                }
                                n570 = And(x=w796, y=w799) -> (x .and. y?=w794:bool)
                                n571 = And(x=w794, y=w800) -> (x .and. y?=w803:bool)
                                n572 = case shown="True" w803 {
                                tunnel: w805 -> [_ w816]
                                frame False {
                                n573 = local write "Temperature Control 5"(FALSE ("Temperature Control 5")) -> ()
                                }
                                frame True {
                                n574 = local write "Temperature SP 5"(w816) -> ()
                                n575 = local write "Temperature Control 5"(TRUE ("Temperature Control 5")) -> ()
                                }
                                }
                                n576 = Wait (ms)(milliseconds to wait=u32 300) -> ()  [unwired: 1 out]
                              }
                            }
                          }
                          frame #1 {
                            # "Wait till Steady State temperature readings on all bays"
                            n577 = while {
                              tunnel: w819 -> [w820]
                              stop <- w821 stop-if-true
                              n578 = flat-sequence {
                                tunnel: [w824] -> w821
                                tunnel: w820 -> [w823]
                                frame #0 {
                                n579 = Wait (ms)(milliseconds to wait=u32 1500) -> ()  [unwired: 1 out]
                                }
                                frame #1 {
                                n580 = local read "Temp SS? 2"() -> (w827:bool)
                                n581 = local read "Temp SS? 3"() -> (w828:bool)
                                n582 = local read "Temp SS? 4"() -> (w829:bool)
                                n583 = local read "Temp SS? 5"() -> (w830:bool)
                                n584 = local read "Temp SS? 1"() -> (w826:bool)
                                n585 = Not(x=w823) -> (.not. x?=w836:bool)
                                n586 = local read "Stop"() -> (w825:bool)
                                n587 = And(x=w828, y=w829) -> (x .and. y?=w832:bool)
                                n588 = And(x=w826, y=w827) -> (x .and. y?=w833:bool)
                                n589 = And(x=w833, y=w832) -> (x .and. y?=w831:bool)
                                n590 = And(x=w831, y=w830) -> (x .and. y?=w834:bool)
                                n591 = Or(x=w836, y=w834) -> (x .or. y?=w835:bool)
                                n592 = Or(x=w835, y=w825) -> (x .or. y?=w824:bool)
                                }
                              }
                            }
                            n593 = local write "Calculate condition"(TRUE ("Calculate condition")) -> ()
                          }
                          frame #2 {
                            n594 = flat-sequence {
                              tunnel: w839 -> [w841]
                              tunnel: [w841] -> w838
                              tunnel: w838 -> [w848]
                              tunnel: [w848] -> w837
                              frame #0 {
                                n595 = local write "Equlibrating Temperature"(TRUE) -> ()
                              }
                              frame #1 {
                                # "Wait 1.5 system volumes"
                                n596 = local read "Number of System Flushes per condtion"() -> (w845:dbl)
                                n597 = local read "Extra system dead volume"() -> (w846:dbl)
                                n598 = script code="start = tic;\nP_tot = P1+P2+P3+P4+P5+P6;\nif P_tot >0\n  extra_res = extr_sys_dead_vol/P_tot;\nelse\n   extra_res =0;\nend\ntotal_sys_res = tau1 + tau2 + tau3 + tau4 + tau5 + extra_res;\ntotal_wait_time = total_sys_res*num_flush_per_cond*60;"("extr_sys_dead_vol"=w846, "num_flush_per_cond"=w845) -> ("??"=w849:errorcluster, "total_wait_time"=w843:dbl, "total_sys_res"=→"Total System Resisdence Time(min)":dbl)  [unwired: 1 in]
                                n599 = Divide(x=w843, y=60.0) -> (x/y=→"total_flush_time":dbl)
                                n600 = while {
                                tunnel: w848 -> [w851]
                                tunnel: w849 -> [w854]
                                stop <- w855 stop-if-true
                                # "Check if system is flushed every 10 seconds"
                                n601 = script code="end1 = toc(start);\nflush_time = 0;\nif end1 > total_wait_time\n   flush_time = 1;\nend\ncurr_wait_time = end1 /60;"("??"=w854) -> ("flush_time"=w858:dbl, "curr_wait_time"=w853:dbl)  [unwired: 1 out]
                                "curr_wait_time" <- w853
                                n602 = Not Equal To 0?(x=w858) -> (x != 0?=w857:bool)
                                n603 = Multiply(x=60.0, y=w853) -> ()  [unwired: 1 out]
                                n604 = local read "Stop"() -> (w860:bool)
                                n605 = Or(x=w857, y=w860) -> (x .or. y?=w856:bool)
                                n606 = Not(x=w851) -> (.not. x?=w850:bool)
                                n607 = Wait (ms)(milliseconds to wait=u32 5000) -> ()  [unwired: 1 out]
                                n608 = Or(x=w856, y=w850) -> (x .or. y?=w855:bool)
                                }
                              }
                            }
                          }
                          frame #3 {
                          }
                          frame #4 {
                            # "Collect HPLC Data"
                            n609 = flat-sequence {
                              tunnel: w864 -> [w873]
                              tunnel: w863 -> [w872]
                              tunnel: w862 -> [w871]
                              tunnel: w862 -> [w870]
                              frame #0 {
                                n610 = local read "pause for ms"() -> (w867:bool)
                                n611 = case shown="True" w867 {
                                frame False {
                                }
                                frame True {
                                n612 = One Button Dialog(message="Press OK to Analyze Data", button name ("OK")="OK" ("Left Button Text (\"Yes\")")) -> ()  [unwired: 1 out]
                                }
                                }
                                n613 = local write "Flushing System"(TRUE ("Flushing System")) -> ()
                                "System Flushed?" <- TRUE ("System Flushed?")
                              }
                              frame #1 {
                                n614 = flat-sequence {
                                tunnel: w873 -> [w878]
                                tunnel: w872 -> [_]
                                tunnel: w871 -> [w877]
                                tunnel: w870 -> [w876]
                                frame #0 {
                                }
                                frame #1 {
                                n615 = flat-sequence {
                                tunnel: w878 -> [w879]
                                tunnel: w878 -> [_]
                                tunnel: [w953] -> w875
                                tunnel: [w952] -> w874
                                tunnel: w876 -> [w951]
                                tunnel: w877 -> [_]
                                tunnel: w874 -> [w965]
                                tunnel: w875 -> [w966]
                                frame #0 {
                                n616 = local read "COMM Port :: Milligat Pumps"() -> (w881:refnum<visa-resource-name>)
                                n617 = stacked-sequence {
                                tunnel: w881 -> [w884 w896 w914 w919 w928 w941]
                                tunnel: w879 -> [w883 w892 w911 w921 w930 w937]
                                tunnel: 1.0 ("Flowrate(ul/min)") -> [w882 w891 w909 w918 w927 w936]
                                frame #0 {
                                n618 = Index Array(array=w883, index=0) -> (element=w886:dbl)
                                n619 = Greater Than 0?(x=w886) -> (x > 0?=w885:bool)
                                n620 = case shown="True" w885 {
                                tunnel: w884 -> [_ w889]
                                tunnel: w882 -> [_ w888]
                                frame False {
                                }
                                frame True {
                                n621 = call "PumpDispense.vi"("Flowrate(ul/min)"=w888, "Pump Address"="j", "Pump COMM Port"=w889) -> ()  [unwired: 7 in, 2 out]
                                }
                                }
                                }
                                frame #1 {
                                n622 = Index Array(array=w892, index=1) -> (element=w894:dbl)
                                n623 = Greater Than 0?(x=w894) -> (x > 0?=w893:bool)
                                n624 = case shown="True" w893 {
                                tunnel: w891 -> [_ w898]
                                tunnel: w896 -> [_ w897]
                                frame False {
                                }
                                frame True {
                                n625 = local read "Syringe_pump?"() -> (w899:bool)
                                n626 = case shown="False" w899 {
                                tunnel: w898 -> [w900 _]
                                tunnel: w897 -> [w901 _]
                                frame False {
                                n627 = call "PumpDispense.vi"("Flowrate(ul/min)"=w900, "Pump Address"="f", "Pump COMM Port"=w901) -> ()  [unwired: 7 in, 2 out]
                                }
                                frame True {
                                w908 = u16 0 items=["Infuse", "Withdraw"] ("Run Direction (0:Infuse)")
                                w904 = u32 4 items=["milliliters per hour (ml/hr)", "milliliters per minute (ml/min)", "milliliters per second (ml/sec)", "microliters per hour (ul/hr)", "microliters per minute (ul/min)", "microliters per second (ul/sec)", "nanoliters per hour (nl/hr)", "nanoliters per minute (nl/min)", "nanoliters per second (nl/sec)", "picoliters per hour (pl/hr)", "picoliters per minute (pl/min)", "picoliters per second (pl/sec)"] ("Flow Rate Units (1:ml/min)")
                                w905 = u16 0 items=["Infuse", "Withdraw"] ("Pump Direction (0:Infuse)")
                                n628 = local read "COMM Port:: Harvard Syringe Pump"() -> (w906:refnum<visa-resource-name>)
                                n629 = call <instrlib>:"Configure Flow Rate & Direction.vi"("VISA resource name"=w906, "Pump Direction (0:Infuse)"=w905, "Flow Rate (5.00)"=i8 2 ("Pump Address"), "Flow Rate Units (1:ml/min)"=w904) -> ("VISA resource name out"=w907:refnum<visa-resource-name>)  [unwired: 10 in, 1 out]
                                n630 = call <instrlib>:"Start Pump.vi"("Run Direction (0:Infuse)"=w908, "VISA resource name"=w907) -> ()  [unwired: 8 in, 2 out]
                                }
                                }
                                }
                                }
                                }
                                frame #2 {
                                n631 = Index Array(array=w911, index=2) -> (element=w912:dbl)
                                n632 = Greater Than 0?(x=w912) -> (x > 0?=w910:bool)
                                n633 = case shown="True" w910 {
                                tunnel: w914 -> [_ w916]
                                tunnel: w909 -> [_ w915]
                                frame False {
                                }
                                frame True {
                                n634 = call "PumpDispense.vi"("Flowrate(ul/min)"=w915, "Pump Address"="i", "Pump COMM Port"=w916) -> ()  [unwired: 7 in, 2 out]
                                }
                                }
                                }
                                frame #3 {
                                n635 = Index Array(array=w921, index=3) -> (element=w922:dbl)
                                n636 = Greater Than 0?(x=w922) -> (x > 0?=w920:bool)
                                n637 = case shown="False" w920 {
                                tunnel: w919 -> [_ w925]
                                tunnel: w918 -> [_ w924]
                                frame False {
                                }
                                frame True {
                                n638 = call "PumpDispense.vi"("Flowrate(ul/min)"=w924, "Pump Address"="g", "Pump COMM Port"=w925) -> ()  [unwired: 7 in, 2 out]
                                }
                                }
                                }
                                frame #4 {
                                n639 = Index Array(array=w930, index=4) -> (element=w931:dbl)
                                n640 = Greater Than 0?(x=w931) -> (x > 0?=w929:bool)
                                n641 = case shown="True" w929 {
                                tunnel: w928 -> [_ w934]
                                tunnel: w927 -> [_ w933]
                                frame False {
                                }
                                frame True {
                                n642 = call "PumpDispense.vi"("Flowrate(ul/min)"=w933, "Pump Address"="e", "Pump COMM Port"=w934) -> ()  [unwired: 7 in, 2 out]
                                }
                                }
                                }
                                frame #5 {
                                n643 = Index Array(array=w937, index=5) -> (element=w939:dbl)
                                n644 = Greater Than 0?(x=w939) -> (x > 0?=w938:bool)
                                n645 = case shown="True" w938 {
                                tunnel: w941 -> [_ w943]
                                tunnel: w936 -> [_ w942]
                                frame False {
                                }
                                frame True {
                                n646 = call "PumpDispense.vi"("Flowrate(ul/min)"=w942, "Pump Address"="h", "Pump COMM Port"=w943) -> ()  [unwired: 7 in, 2 out]
                                }
                                }
                                }
                                }
                                }
                                frame #1 {
                                n647 = while {
                                stop <- w950 stop-if-true
                                n648 = local read "Phase_Sensor_voltage"() -> (w945:dbl)
                                n649 = script code="organic_phase = 0;\nif start_phase_time \n   start_phase_timer = tic;\n   start_phase_time = 0;\nelse\n  %ignore phase sensor values\n  %if not(phase_sensor_val >2.9 && phase_sensor_val <3.8)\n    %    start_phase_timer = tic;\n   %end\n\n   end_phase_time =  toc(start_phase_timer )\n\n   if end_phase_time > 2\n       organic_phase = 1;\n       start_phase_time = 1;\n   end\n\nend"("phase_sensor_val"=w945) -> ("organic_phase"=w947:dbl)  [unwired: 1 in, 1 out]
                                n650 = local read "Stop"() -> (w949:bool)
                                n651 = Not Equal To 0?(x=w947) -> (x != 0?=w948:bool)
                                n652 = Or(x=w948, y=w949) -> (x .or. y?=w950:bool)
                                n653 = Wait (ms)(milliseconds to wait=u32 300) -> ()  [unwired: 1 out]
                                }
                                }
                                frame #2 {
                                n654 = local read "Stop"() -> (w955:bool)
                                n655 = local read "Bay Parameters"() -> (w952:T2)
                                n656 = Not(x=w955) -> (.not. x?=w954:bool)
                                n657 = case shown="True" w954 {
                                tunnel: [errorcluster {"status"=FALSE, "code"=0, "source"=""} ("error out") w959] -> w953
                                tunnel: w952 -> [_ w958]
                                tunnel: w951 -> [_ w957]
                                frame False {
                                }
                                frame True {
                                n658 = flat-sequence {
                                tunnel: [w962] -> w959
                                tunnel: w958 -> [w964]
                                tunnel: w957 -> [_]
                                frame #0 {
                                n659 = Wait (ms)(milliseconds to wait=u32 15000) -> ()  [unwired: 1 out]
                                }
                                frame #1 {
                                # "Read Raman Data"
                                n660 = Unbundle By Name(w964) -> ("Raman File Name"=w963:string)
                                n661 = call "Raman_READ_WRITE.vi"("Number of files to read"=1.0, "IR Read Dir."=w963) -> ("error constant 2"=w962:errorcluster)  [unwired: 6 in, 3 out]
                                }
                                }
                                }
                                }
                                }
                                frame #3 {
                                n662 = Unbundle By Name(w966) -> ("status"=w967:bool)
                                n663 = case shown="True" w967 {
                                tunnel: w965 -> [_ w968]
                                frame False {
                                }
                                frame True {
                                n664 = while {
                                tunnel: w968 -> [w970]
                                stop <- w969 stop-if-true
                                w975 = "An error occured while trying to read Raman data. " ("message")
                                n665 = local write "Error Message"(w975) -> ()
                                n666 = call <vilib>:"Three Button Dialog.vi"("Right Button Text (\"Cancel\")"="STOP EXPs" ("F button name (\"Cancel\")"), "Center Button Text (\"No\")"="REDO" ("T button name (\"OK\")"), "Left Button Text (\"Yes\")"="REREAD" ("T button name (\"OK\")"), "message"=w975) -> ("Which Button?"=w971:T19)  [unwired: 7 in]
                                n667 = case shown="\"Left Button\"" w971 {
                                tunnel: w970 -> [_ _ w984 _]
                                tunnel: [TRUE TRUE w983 w985] -> w969
                                frame "Right Button" {
                                w976 = TRUE ("Setup Error")
                                n668 = local write "System Error"(w976) -> ()
                                n669 = local write "Setup Error"(w976) -> ()
                                n670 = script code="system_error = 1"() -> ()  [unwired: 1 in, 1 out]
                                n671 = local write "Stop"(w976) -> ()
                                }
                                frame "Center Button" {
                                n672 = script code="redo = true;\nopt_ctr = 1;\nCurrExp = CurrExp + 1;\nncall0 = ncall0 +1;\nif req_ctr == req_tot\n       opt_ctr = 3;\n  else\n     req_ctr = req_ctr +1;\nend"() -> ()  [unwired: 1 in, 1 out]
                                }
                                frame "Left Button" {
                                n673 = Unbundle By Name(w984) -> ("Raman File Name"=w980:string)
                                n674 = call "Raman_READ_WRITE.vi"("Number of files to read"=1.0, "IR Read Dir."=w980) -> ("error constant 2"=w981:errorcluster)  [unwired: 6 in, 3 out]
                                n675 = Unbundle By Name(w981) -> ("status"=w982:bool)
                                n676 = Not(x=w982) -> (.not. x?=w983:bool)
                                }
                                frame "Window Close" {
                                w985 = TRUE
                                n677 = local write "Setup Error"(w985) -> ()
                                n678 = script code="system_error = 1"() -> ()  [unwired: 1 in, 1 out]
                                n679 = local write "Stop"(w985) -> ()
                                }
                                }
                                }
                                }
                                }
                                }
                                }
                                }
                                }
                              }
                              frame #2 {
                                n680 = local read "Stop"() -> (w987:bool)
                                n681 = local write "HPLC Analysis"(TRUE ("HPLC Analysis")) -> ()
                                n682 = Not(x=w987) -> (.not. x?=w986:bool)
                                n683 = case shown="True" w986 {
                                frame False {
                                }
                                frame True {
                                n684 = script code="C_measured =product;\nConc = product;\nFvalues(end +1,:) = [product];"() -> ()  [unwired: 1 in, 1 out]
                                }
                                }
                              }
                            }
                          }
                          frame #5 {
                            n685 = local read "Stop"() -> (w990:bool)
                            n686 = Not(x=w990) -> (.not. x?=w989:bool)
                            n687 = case shown="True" w989 {
                              tunnel: [1.0 w1001] -> w991
                              frame False {
                              }
                              frame True {
                                # "Save data to excel file"
                                n688 = local read "Bay Parameters"() -> (w999:T2)
                                n689 = Unbundle By Name(w999) -> ("Total Number of Experiments 2"=w998:dbl)
                                n690 = script code="analyze_labview_results"("ncall"=w998) -> ("terminate"=w1001:dbl, "ncall0"=w1000:dbl, "experiment_history"=w996:dbl[][], "Pbest"=w994:dbl[], "Tbest"=w995:dbl[], "best_exp_num"=w993:dbl)  [unwired: 1 in, 1 out]
                                n691 = local write "Flowrates(ul/min)_best"(w994) -> ()
                                n692 = local write "temperature_best"(w995) -> ()
                                n693 = local write "best_exp_num"(w993) -> ()
                                n694 = local write "Current Experiment"(w1000) -> ()
                                n695 = local write "Total Number of Experiments"(w998) -> ()
                                n696 = call-poly <vilib>:"Array To Matrix.vi"("Real 2D Array"=w996) -> ("Real Matrix"=w997:T18)
                                n697 = local write "experiment history"(w997) -> ()
                              }
                            }
                          }
                          frame #6 {
                            n698 = local read "Num_exp_till_pause"() -> (w1003:i32)
                            n699 = Increment(x=w1003) -> (x+1=w1002:i32)
                            n700 = local write "Num_exp_till_pause"(w1002) -> ()
                          }
                          frame #7 {
                            # "Pause System"
                            n701 = local read "Bay Parameters"() -> (w1011:T2)
                            n702 = Unbundle By Name(w1011) -> ("Num_conditons_per_wait"=w1010:dbl)
                            n703 = local read "Num_exp_till_pause"() -> (w1009:i32)
                            n704 = Equal?(x=w1010, y=w1009) -> (x = y?=w1008:bool)
                            n705 = local read "Run_Stop_cluster"() -> (w1005:T7)
                            n706 = Unbundle By Name(w1005) -> ("Stop Run Button"=w1007:bool)
                            n707 = Or(x=w1007, y=w1008) -> (x .or. y?=w1006:bool)
                            n708 = case shown="True" w1006 {
                              tunnel: w1010 -> [w1014 _]
                              tunnel: w1009 -> [w1015 _]
                              tunnel: w1005 -> [_ w1017]
                              frame False {
                                n709 = Greater?(x=w1015, y=w1014) -> (0:w1013:bool)
                                n710 = case shown="True" w1013 {
                                frame False {
                                }
                                frame True {
                                n711 = local write "Num_exp_till_pause"(0 ("Num_exp_till_pause")) -> ()
                                }
                                }
                              }
                              frame True {
                                n712 = flat-sequence {
                                tunnel: w1017 -> [w1045]
                                frame #0 {
                                w1021 = string[] ["e", "f", "g", "h", "i", "j"]
                                # "Turn off pumps and stop controling temperature"
                                n713 = stacked-sequence {
                                frame #0 {
                                n714 = local write "Temperature Control 1"(FALSE ("Temperature Control 1")) -> ()
                                }
                                frame #1 {
                                n715 = local write "Temperature Control 2"(FALSE ("Temperature Control 2")) -> ()
                                }
                                frame #2 {
                                n716 = local write "Temperature Control 3"(FALSE ("Temperature Control 3")) -> ()
                                }
                                frame #3 {
                                n717 = local write "Temperature Control 4"(FALSE ("Temperature Control 4")) -> ()
                                }
                                frame #4 {
                                n718 = local write "Temperature Control 5"(FALSE ("Temperature Control 5")) -> ()
                                }
                                }
                                n719 = local read "COMM Port:: Harvard Syringe Pump"() -> (w1019:refnum<visa-resource-name>)
                                n720 = local read "Syringe_pump?"() -> (w1018:bool)
                                n721 = local read "COMM Port :: Milligat Pumps"() -> (w1020:refnum<visa-resource-name>)
                                n722 = Array Size(array=w1021) -> (size(s)=w1022:i32)
                                n723 = case shown="True" w1018 {
                                tunnel: w1019 -> [_ w1030]
                                frame False {
                                }
                                frame True {
                                n724 = call <instrlib>:"Stop Pump.vi"("VISA resource name"=w1030) -> ()  [unwired: 9 in, 2 out]
                                }
                                }
                                n725 = for {
                                N: w1022 -> [_]
                                tunnel: w1021 -> [w1028] mode=indexing
                                tunnel: w1020 -> [w1029]
                                n726 = call "PumpStop.vi"("Pump Address"=w1028, "Pump COMM Port"=w1029) -> ()  [unwired: 9 in, 1 out]
                                }
                                }
                                frame #1 {
                                n727 = local read "Stop"() -> (w1033:bool)
                                n728 = Not(x=w1033) -> (.not. x?=w1032:bool)
                                n729 = case shown="True" w1032 {
                                frame False {
                                }
                                frame True {
                                n730 = while {
                                stop <- w1039 stop-if-true
                                # "Wait till user confirms system resume"
                                n731 = Two Button Dialog(message="System is currently paused. Refill Syringes, flush lines, then press OK to continue optimization.\nOr Redo to repeat condition ", 1:"REDO" ("F button name (\"Cancel\")"), 2:"OK" ("Left Button Text (\"Yes\")")) -> (T button?=w1035:bool)
                                n732 = case shown="False" w1035 {
                                tunnel: [TRUE TRUE] -> w1034
                                frame False {
                                n733 = script code="redo = true;"() -> ()  [unwired: 1 in, 1 out]
                                }
                                frame True {
                                }
                                }
                                n734 = local read "Stop"() -> (w1040:bool)
                                n735 = Or(x=w1034, y=w1040) -> (x .or. y?=w1039:bool)
                                }
                                }
                                }
                                n736 = local write "stop_xl_write"(TRUE ("stop_xl_write")) -> ()
                                }
                                frame #2 {
                                n737 = local write "Num_exp_till_pause"(0 ("Num_exp_till_pause")) -> ()
                                n738 = Bundle By Name(cluster=w1045, "Stop Run Button"=FALSE) -> (w1043:T7)
                                n739 = local write "Run_Stop_cluster"(w1043) -> ()
                                }
                                }
                              }
                            }
                          }
                          frame #8 {
                            w1048 = FALSE
                            n740 = local write "Equlibrating Temperature"(w1048) -> ()
                            n741 = local write "Calculate condition"(w1048) -> ()
                            n742 = local write "Flushing System"(w1048) -> ()
                            n743 = local write "HPLC Analysis"(w1048) -> ()
                            n744 = local write "stop_xl_write"(TRUE ("stop_xl_write")) -> ()
                          }
                        }
                        n745 = while {
                          stop <- w1075 stop-if-true
                          n746 = flat-sequence {
                            frame #0 {
                              n747 = script code="save_excel_time_data;"() -> ()  [unwired: 1 in, 1 out]
                            }
                            frame #1 {
                              n748 = Wait (ms)(milliseconds to wait=u32 30000) -> ()  [unwired: 1 out]
                            }
                          }
                          n749 = local read "Stop"() -> (w1076:bool)
                          n750 = local read "stop_xl_write"() -> (w1074:bool)
                          n751 = Or(x=w1074, y=w1076) -> (x .or. y?=w1075:bool)
                        }
                      }
                    }
                  }
                }
                n752 = Greater?(x=w602, y=w603) -> (0:w610:bool)
                n753 = Equal?(x=w608, y=1.0) -> (x = y?=w604:bool)
                n754 = local read "Stop"() -> (w611:bool)
                n755 = Or(x=w611, y=w610) -> (x .or. y?=w607:bool)
                n756 = Or(x=w604, y=w607) -> (x .or. y?=w606:bool)
                n757 = case shown="True" w604 {
                  frame False {
                  }
                  frame True {
                    w615 = u16 2 items=["System  Error", "System Running", "System Standby"] ("System Status")
                    n758 = local write "Stop"(TRUE ("Stop")) -> ()
                    n759 = local write "System Status"(w615) -> ()
                  }
                }
                "Optimization_loop_index" <- w612
              }
            }
          }
          n760 = while {
            tunnel: w590 -> [w1171]
            stop <- w1174 stop-if-true
            n761 = local read "Temperature Control 3"() -> (w1172:bool)
            n762 = local read "running?"() -> (w1170:bool)
            n763 = And(x=w1170, y=w1172) -> (x .and. y?=w1173:bool)
            n764 = case shown="True" w1173 {
              tunnel: w1171 -> [_ w1177]
              frame False {
                n765 = local write "Temp SS? 3"(TRUE) -> ()
              }
              frame True {
                # "Bay 3 Temperature Controller"
                n766 = local read "Temperature SP 3"() -> (w1178:dbl)
                n767 = local read "Temperature 3"() -> (w1181:dbl)
                n768 = Subtract(x=w1181, y=w1178) -> (x-y=w1190:dbl)
                n769 = Absolute Value(x=w1190) -> (abs(x)=w1192:dbl)
                n770 = Less Or Equal?(x=w1192, y=1.2) -> (x <= y?=w1189:bool)
                n771 = local write "Temp SS? 3"(w1189) -> ()
                n772 = local read "SSR Duration 3"() -> (w1199:dbl)
                n773 = call-poly <vilib>:"PID Online Autotuning.vi"("setpoint"=w1178, "manipulated variable"=w1199, "autotuning parameters"=T9 {"type of controller"=enum."PID", "relay cycles"=3, "relay amplitude"=1.0, "control specifications"=enum."Normal", "PV noise level"=0.1} ("Autotuning Parameters R1"), "process variable"=w1181, "PID gains in"=T8 {"Proportional gain Kc"=0.38538, "Integral time Ti (sec)"=0.524375, "Derivative time Ti (sec)"=0.12585} ("PID gains 2")) -> ("setpoint out"=w1197:dbl, "process variable out"=w1198:dbl, "PID gains out"=w1201:T17)  [unwired: 6 in, 2 out]
                n774 = Greater?(x=w1178, y=w1181) -> (0:w1188:bool)
                n775 = call <vilib>:"PID Autotuning (Temperature).vi"("desired temperature"=w1197, "measured temperature"=w1198, "PID gains in"=w1201, "output range"=cluster{"output high":dbl, "output low":dbl} {"output high"=3.0, "output low"=-1.0} ("Output range")) -> ("output"=w1194:dbl)  [unwired: 12 in, 3 out]
                n776 = Multiply(x=1000.0, y=w1194) -> (x*y=w1196:dbl)
                n777 = local write "SSR Duration 3"(w1194) -> ()
                n778 = Greater Than 0?(x=w1196) -> (x > 0?=w1187:bool)
                n779 = And(x=w1187, y=w1188) -> (x .and. y?=w1185:bool)
                n780 = Subtract(x=w1181, y=10.0) -> (x-y=w1183:dbl)
                n781 = Less?(x=w1183, y=w1178) -> (x < y?=w1186:bool)
                n782 = And(x=w1186, y=w1185) -> (x .and. y?=w1184:bool)
                n783 = case shown="True" w1184 {
                  tunnel: [errorcluster {"status"=FALSE, "code"=0, "source"=""} ("error out") w1213] -> _
                  tunnel: 4 -> [_ w1211]
                  tunnel: w1196 -> [w1207 w1212]
                  tunnel: [0.0 w1215] -> w1179
                  tunnel: w1178 -> [_ w1214]
                  tunnel: w1177 -> [_ w1210]
                  frame False {
                    n784 = Absolute Value(x=w1207) -> (abs(x)=w1208:dbl)
                    n785 = Wait (ms)(milliseconds to wait=w1208) -> ()  [unwired: 1 out]
                  }
                  frame True {
                    n786 = call "TurnOnRelayArduino.vi"("channel"=w1211, "duration"=w1212, "LINX Resource"=w1210) -> ("error out"=w1213:errorcluster)  [unwired: 7 in, 1 out]
                    n787 = script code="tempdiff3= SP3 - T3;\nif tempdiff3 > 10\n  if slope3 < .01\n     temp_check3 = temp_check3 + 1;\n  else\n      temp_check3 =0;\n  end\nend\n\nif temp_check3 > 9\n  temp_error3 = 1\nend"("SP3"=w1214) -> ("temp_error3"=w1215:dbl)  [unwired: 1 in, 1 out]
                  }
                }
                n788 = Not Equal To 0?(x=w1179) -> (x != 0?=w1180:bool)
                n789 = case shown="True" w1180 {
                  frame False {
                  }
                  frame True {
                    n790 = local write "Error Message"("Bay 3 Temperature Heating Error") -> ()
                  }
                }
                n791 = case shown="True" w1180 {
                  tunnel: w1180 -> [_ w1205]
                  frame False {
                  }
                  frame True {
                    n792 = local write "System Error"(w1205) -> ()
                    n793 = local write "Stop"(w1205) -> ()
                  }
                }
              }
            }
            n794 = Wait (ms)(milliseconds to wait=u32 400) -> ()  [unwired: 1 out]
            n795 = local read "Stop"() -> (w1174:bool)
          }
          n796 = while {
            tunnel: w590 -> [w1125]
            stop <- w1128 stop-if-true
            n797 = local read "running?"() -> (w1124:bool)
            n798 = Wait (ms)(milliseconds to wait=u32 400) -> ()  [unwired: 1 out]
            n799 = local read "Temperature Control 4"() -> (w1127:bool)
            n800 = And(x=w1124, y=w1127) -> (x .and. y?=w1126:bool)
            n801 = case shown="True" w1126 {
              tunnel: w1125 -> [_ w1131]
              frame False {
                n802 = local write "Temp SS? 4"(TRUE ("Temp SS? 4")) -> ()
              }
              frame True {
                # "Bay 4 Temperature Controller"
                n803 = local read "Temperature SP 4"() -> (w1134:dbl)
                n804 = local read "Temperature 4"() -> (w1137:dbl)
                n805 = Subtract(x=w1137, y=w1134) -> (x-y=w1144:dbl)
                n806 = Absolute Value(x=w1144) -> (abs(x)=w1146:dbl)
                n807 = Less Or Equal?(x=w1146, y=1.2) -> (x <= y?=w1143:bool)
                n808 = local write "Temp SS? 4"(w1143) -> ()
                n809 = local read "SSR Duration 4"() -> (w1147:dbl)
                n810 = call-poly <vilib>:"PID Online Autotuning.vi"("setpoint"=w1134, "manipulated variable"=w1147, "autotuning parameters"=T9 {"type of controller"=enum."PID", "relay cycles"=3, "relay amplitude"=1.0, "control specifications"=enum."Normal", "PV noise level"=0.1} ("Autotuning Parameters R1"), "process variable"=w1137, "PID gains in"=T8 {"Proportional gain Kc"=0.38538, "Integral time Ti (sec)"=0.524375, "Derivative time Ti (sec)"=0.12585} ("PID gains 2")) -> ("setpoint out"=w1149:dbl, "process variable out"=w1150:dbl, "PID gains out"=w1152:T17)  [unwired: 6 in, 2 out]
                n811 = call <vilib>:"PID Autotuning (Temperature).vi"("desired temperature"=w1149, "measured temperature"=w1150, "PID gains in"=w1152, "output range"=cluster{"output high":dbl, "output low":dbl} {"output high"=3.0, "output low"=-1.0} ("Output range")) -> ("output"=w1148:dbl)  [unwired: 12 in, 3 out]
                n812 = Subtract(x=w1137, y=10.0) -> (x-y=w1136:dbl)
                n813 = Less?(x=w1136, y=w1134) -> (x < y?=w1138:bool)
                n814 = Multiply(x=1000.0, y=w1148) -> (x*y=w1156:dbl)
                n815 = Greater?(x=w1134, y=w1137) -> (0:w1142:bool)
                n816 = Greater Than 0?(x=w1156) -> (x > 0?=w1141:bool)
                n817 = local write "SSR Duration 4"(w1148) -> ()
                n818 = And(x=w1141, y=w1142) -> (x .and. y?=w1140:bool)
                n819 = And(x=w1138, y=w1140) -> (x .and. y?=w1139:bool)
                n820 = case shown="True" w1139 {
                  tunnel: [errorcluster {"status"=FALSE, "code"=0, "source"=""} ("error out") w1167] -> _
                  tunnel: 5 -> [_ w1165]
                  tunnel: w1156 -> [w1161 w1166]
                  tunnel: w1134 -> [_ w1169]
                  tunnel: [0.0 w1168] -> w1133
                  tunnel: w1131 -> [_ w1164]
                  frame False {
                    n821 = Absolute Value(x=w1161) -> (abs(x)=w1162:dbl)
                    n822 = Wait (ms)(milliseconds to wait=w1162) -> ()  [unwired: 1 out]
                  }
                  frame True {
                    n823 = call "TurnOnRelayArduino.vi"("channel"=w1165, "duration"=w1166, "LINX Resource"=w1164) -> ("error out"=w1167:errorcluster)  [unwired: 7 in, 1 out]
                    n824 = script code="tempdiff4= SP4 - T4;\nif tempdiff4 > 10\n  if slope4 < .01\n     temp_check4 = temp_check4 + 1;\n  else\n      temp_check4 =0;\n  end\nend\n\nif temp_check4 > 9\n  temp_error4 = 1\nend"("SP4"=w1169) -> ("temp_error4"=w1168:dbl)  [unwired: 1 in, 1 out]
                  }
                }
                n825 = Not Equal To 0?(x=w1133) -> (x != 0?=w1132:bool)
                n826 = case shown="True" w1132 {
                  frame False {
                  }
                  frame True {
                    n827 = local write "Error Message"("Bay 4 Temperature Heating Error") -> ()
                  }
                }
                n828 = case shown="True" w1132 {
                  tunnel: w1132 -> [_ w1159]
                  frame False {
                  }
                  frame True {
                    n829 = local write "System Error"(w1159) -> ()
                    n830 = local write "Stop"(w1159) -> ()
                  }
                }
              }
            }
            n831 = local read "Stop"() -> (w1128:bool)
          }
          n832 = while {
            stop <- w595 stop-if-true
            n833 = script code="TempArr1=circshift(TempArr1,9);\nTempArr2=circshift(TempArr2,9);\nTempArr3=circshift(TempArr3,9);\nTempArr4=circshift(TempArr4,9);\nTempArr5=circshift(TempArr5,9);\n\nTempArr1(10)=T1;\nTempArr2(10)=T2;\nTempArr3(10)=T3;\nTempArr4(10)=T4;\nTempArr5(10)=T5;\n\n[slope1 temp] = polyfit([1,2,3,4,5,6,7,8,9,10]',TempArr1,1);\nslope1 = slope1(1);\n[slope2 temp] = polyfit([1,2,3,4,5,6,7,8,9,10]',TempArr2,1);\nslope2= slope2(1);\n[slope3 temp] = polyfit([1,2,3,4,5,6,7,8,9,10]',TempArr3,1);\nslope3 = slope3(1);\n[slope4 temp] = polyfit([1,2,3,4,5,6,7,8,9,10]',TempArr4,1);\nslope4 = slope4(1);\n[slope5 temp] = polyfit([1,2,3,4,5,6,7,8,9,10]',TempArr5,1);\nslope5 = slope5(1);"() -> ()  [unwired: 1 in, 1 out]
            n834 = Wait (ms)(milliseconds to wait=u32 600) -> ()  [unwired: 1 out]
            n835 = local read "Stop"() -> (w595:bool)
          }
          n836 = while {
            tunnel: w590 -> [w1079]
            stop <- w1082 stop-if-true
            n837 = local read "running?"() -> (w1078:bool)
            n838 = local read "Temperature Control 5"() -> (w1080:bool)
            n839 = And(x=w1078, y=w1080) -> (x .and. y?=w1081:bool)
            n840 = case shown="True" w1081 {
              tunnel: w1079 -> [_ w1085]
              frame False {
                n841 = local write "Temp SS? 5"(TRUE ("Temp SS? 5")) -> ()
              }
              frame True {
                # "Bay 5 Temperature Controller"
                n842 = local read "SSR Duration 5"() -> (w1101:dbl)
                n843 = local read "Temperature SP 5"() -> (w1087:dbl)
                n844 = local read "Temperature 5"() -> (w1090:dbl)
                n845 = Subtract(x=w1090, y=w1087) -> (x-y=w1098:dbl)
                n846 = Absolute Value(x=w1098) -> (abs(x)=w1100:dbl)
                n847 = Less Or Equal?(x=w1100, y=1.2) -> (x <= y?=w1097:bool)
                n848 = local write "Temp SS? 5"(w1097) -> ()
                n849 = call-poly <vilib>:"PID Online Autotuning.vi"("setpoint"=w1087, "manipulated variable"=w1101, "autotuning parameters"=T9 {"type of controller"=enum."PID", "relay cycles"=3, "relay amplitude"=1.0, "control specifications"=enum."Normal", "PV noise level"=0.1} ("Autotuning Parameters R1"), "process variable"=w1090, "PID gains in"=T8 {"Proportional gain Kc"=0.38538, "Integral time Ti (sec)"=0.524375, "Derivative time Ti (sec)"=0.12585} ("PID gains 2")) -> ("setpoint out"=w1103:dbl, "process variable out"=w1104:dbl, "PID gains out"=w1106:T17)  [unwired: 6 in, 2 out]
                n850 = call <vilib>:"PID Autotuning (Temperature).vi"("desired temperature"=w1103, "measured temperature"=w1104, "PID gains in"=w1106, "output range"=cluster{"output high":dbl, "output low":dbl} {"output high"=3.0, "output low"=-1.0} ("Output range")) -> ("output"=w1102:dbl)  [unwired: 12 in, 3 out]
                n851 = Multiply(x=1000.0, y=w1102) -> (x*y=w1110:dbl)
                n852 = Greater?(x=w1087, y=w1090) -> (0:w1095:bool)
                n853 = Greater Than 0?(x=w1110) -> (x > 0?=w1096:bool)
                n854 = local write "SSR Duration 5"(w1102) -> ()
                n855 = And(x=w1096, y=w1095) -> (x .and. y?=w1093:bool)
                n856 = Subtract(x=w1090, y=10.0) -> (x-y=w1091:dbl)
                n857 = Greater?(x=w1091, y=w1087) -> (0:w1094:bool)
                n858 = And(x=w1094, y=w1093) -> (x .and. y?=w1092:bool)
                n859 = case shown="True" w1092 {
                  tunnel: [errorcluster {"status"=FALSE, "code"=0, "source"=""} ("error out") w1121] -> _
                  tunnel: 6 -> [_ w1118]
                  tunnel: w1110 -> [w1115 w1119]
                  tunnel: [0.0 w1123] -> w1088
                  tunnel: w1087 -> [_ w1122]
                  tunnel: w1085 -> [_ w1120]
                  frame False {
                    n860 = Absolute Value(x=w1115) -> (abs(x)=w1116:dbl)
                    n861 = Wait (ms)(milliseconds to wait=w1116) -> ()  [unwired: 1 out]
                  }
                  frame True {
                    n862 = call "TurnOnRelayArduino.vi"("channel"=w1118, "duration"=w1119, "LINX Resource"=w1120) -> ("error out"=w1121:errorcluster)  [unwired: 7 in, 1 out]
                    n863 = script code="tempdiff5= SP5 - T5;\n\nif tempdiff5 > 10\n  if slope5 < .01\n     temp_check5 = temp_check5 + 1;\n  else\n      temp_check5 =0;\n  end\nend\n\nif temp_check5 >9\n  temp_error5 = 1\nend"("SP5"=w1122) -> ("temp_error5"=w1123:dbl)  [unwired: 1 in, 1 out]
                  }
                }
                n864 = Not Equal To 0?(x=w1088) -> (x != 0?=w1086:bool)
                n865 = case shown="True" w1086 {
                  frame False {
                  }
                  frame True {
                    n866 = local write "Error Message"("Bay 5 Temperature Heating Error") -> ()
                  }
                }
                n867 = case shown="True" w1086 {
                  tunnel: w1086 -> [_ w1113]
                  frame False {
                  }
                  frame True {
                    n868 = local write "Stop"(w1113) -> ()
                    n869 = local write "System Error"(w1113) -> ()
                  }
                }
              }
            }
            n870 = Wait (ms)(milliseconds to wait=u32 400) -> ()  [unwired: 1 out]
            n871 = local read "Stop"() -> (w1082:bool)
          }
        }
      }
      n872 = local read "IR Sensor Device"() -> (w62:T6)
      n873 = while {
        tunnel: errorcluster {"status"=FALSE, "code"=0, "source"=""} ("error out") -> [w133]
        tunnel: w62 -> [w152]
        stop <- w173 stop-if-true
        w130 = u8 7 items=["RAM IR raw  Ch1"=4, "RAM IR raw  Ch2"=5, "RAM T_A"=6, "RAM T_OBJ1"=7, "RAM T_OBJ2"=8, "EEPROM_To_max"=32, "EEPROM_To_min"=33, "EEPROM_PWM_CTRL"=34, "EEPROM_Ta_range"=35, "EEPROM_Emissivity_CorrCoeff"=36, "EEPROM_SMBus Address"=46, "EEPROM_ConfigReg"=37] ("Melexis_Cmmds")
        # "Bay 5 Temperature Read"
        # "Bay 4 Temperature Read"
        # "Bay 3 Temperature Read"
        # "Bay 2 Temperature Read"
        # "Bay 1 Temperature Read"
        n874 = local read "Stop"() -> (w173:bool)
        n875 = call "IRSensorNIRead.vi"("error in (no error)"=w133, "Melexis_Cmmds"=w130, "Address"=u8 1, "device reference"=w152) -> ("error out"=w155:errorcluster, "Temperature"=w153:dbl, "device reference out"=w151:T6)  [unwired: 5 in]
        n876 = local write "error out"(w155) -> ()
        n877 = Unbundle By Name(w155) -> ("status"=w154:bool)
        n878 = call-poly <vilib>:"PID Control Input Filter.vi"("input"=w153) -> ("output"=w166:dbl)  [unwired: 4 in]
        n879 = case shown="False" w154 {
          tunnel: w165 -> [w182 _]
          tunnel: [w182 w183] -> w170
          frame False {
            n880 = local write "Temperature 1"(w182) -> ()
          }
          frame True {
            n881 = local read "Temperature 1"() -> (w183:dbl)
          }
        }
        n882 = flat-sequence {
          tunnel: w166 -> [w196]
          tunnel: [w196] -> w165
          tunnel: w151 -> [w195]
          tunnel: [w195] -> w150
          frame #0 {
            n883 = Wait (ms)(milliseconds to wait=u32 100) -> ()  [unwired: 1 out]
          }
        }
        n884 = call "IRSensorNIRead.vi"("error in (no error)"=w133, "Melexis_Cmmds"=w130, "Address"=u8 2, "device reference"=w150) -> ("error out"=w142:errorcluster, "Temperature"=w143:dbl, "device reference out"=w145:T6)  [unwired: 5 in]
        n885 = local write "error out"(w142) -> ()
        n886 = Unbundle By Name(w142) -> ("status"=w147:bool)
        n887 = call-poly <vilib>:"PID Control Input Filter.vi"("input"=w143) -> ("output"=w164:dbl)  [unwired: 4 in]
        n888 = case shown="True" w147 {
          tunnel: w163 -> [w180 _]
          tunnel: [w180 w181] -> w169
          frame False {
            n889 = local write "Temperature 2"(w180) -> ()
          }
          frame True {
            n890 = local read "Temperature 2"() -> (w181:dbl)
          }
        }
        n891 = flat-sequence {
          tunnel: w164 -> [w193]
          tunnel: [w193] -> w163
          tunnel: w145 -> [w192]
          tunnel: [w192] -> w144
          frame #0 {
            n892 = Wait (ms)(milliseconds to wait=u32 100) -> ()  [unwired: 1 out]
          }
        }
        n893 = call "IRSensorNIRead.vi"("error in (no error)"=w133, "Melexis_Cmmds"=w130, "Address"=u8 3, "device reference"=w144) -> ("error out"=w135:errorcluster, "Temperature"=w141:dbl, "device reference out"=w140:T6)  [unwired: 5 in]
        n894 = local write "error out"(w135) -> ()
        n895 = Unbundle By Name(w135) -> ("status"=w136:bool)
        n896 = case shown="False" w136 {
          tunnel: w160 -> [w178 _]
          tunnel: [w178 w179] -> w162
          frame False {
            n897 = local write "Temperature 3"(w178) -> ()
          }
          frame True {
            n898 = local read "Temperature 3"() -> (w179:dbl)
          }
        }
        n899 = call-poly <vilib>:"PID Control Input Filter.vi"("input"=w141) -> ("output"=w161:dbl)  [unwired: 4 in]
        n900 = flat-sequence {
          tunnel: w161 -> [w190]
          tunnel: [w190] -> w160
          tunnel: w140 -> [w189]
          tunnel: [w189] -> w138
          frame #0 {
            n901 = Wait (ms)(milliseconds to wait=u32 100) -> ()  [unwired: 1 out]
          }
        }
        n902 = call "IRSensorNIRead.vi"("error in (no error)"=w133, "Melexis_Cmmds"=w130, "Address"=u8 4, "device reference"=w138) -> ("error out"=w125:errorcluster, "Temperature"=w137:dbl, "device reference out"=w132:T6)  [unwired: 5 in]
        n903 = local write "error out"(w125) -> ()
        n904 = Unbundle By Name(w125) -> ("status"=w127:bool)
        n905 = case shown="True" w127 {
          tunnel: w158 -> [w176 _]
          tunnel: [w176 w177] -> w168
          frame False {
            n906 = local write "Temperature 4"(w176) -> ()
          }
          frame True {
            n907 = local read "Temperature 4"() -> (w177:dbl)
          }
        }
        n908 = call-poly <vilib>:"PID Control Input Filter.vi"("input"=w137) -> ("output"=w159:dbl)  [unwired: 4 in]
        n909 = flat-sequence {
          tunnel: w159 -> [w187]
          tunnel: [w187] -> w158
          tunnel: w132 -> [w186]
          tunnel: [w186] -> w131
          frame #0 {
            n910 = Wait (ms)(milliseconds to wait=u32 100) -> ()  [unwired: 1 out]
          }
        }
        n911 = call "IRSensorNIRead.vi"("error in (no error)"=w133, "Melexis_Cmmds"=w130, "Address"=u8 5, "device reference"=w131) -> ("error out"=w128:errorcluster, "Temperature"=w129:dbl)  [unwired: 5 in, 1 out]
        n912 = local write "error out"(w128) -> ()
        n913 = flat-sequence {
          tunnel: w157 -> [w184]
          tunnel: [w184] -> w156
          frame #0 {
            n914 = Wait (ms)(milliseconds to wait=u32 100) -> ()  [unwired: 1 out]
          }
        }
        n915 = Unbundle By Name(w128) -> ("status"=w126:bool)
        n916 = call-poly <vilib>:"PID Control Input Filter.vi"("input"=w129) -> ("output"=w157:dbl)  [unwired: 4 in]
        n917 = local write "error out"(w133) -> ()
        n918 = Build Array(w170, w169, w162, w168, w156) -> (w172:dbl[])
        n919 = Array To Cluster(array=w172) -> (cluster=→"Teperature Chart":T3)
        n920 = case shown="False" w126 {
          tunnel: w156 -> [w174 _]
          tunnel: [w174 w175] -> w167
          frame False {
            n921 = local write "Temperature 5"(w174) -> ()
          }
          frame True {
            n922 = local read "Temperature 5"() -> (w175:dbl)
          }
        }
        n923 = script code="MATLAB script"("T1"=w170, "T2"=w169, "T3"=w162, "T4"=w168, "T5"=w167) -> ()  [unwired: 1 in, 1 out]
      }
      n924 = while {
        stop <- w88 stop-if-true
        n925 = local read "Pump setpoint(ul/min) 1"() -> (w91:dbl)
        n926 = local read "Pump setpoint(ul/min) 2"() -> (w87:dbl)
        n927 = local read "Pump setpoint(ul/min) 3"() -> (w86:dbl)
        n928 = local read "Pump setpoint(ul/min) 4"() -> (w85:dbl)
        n929 = local read "Pump setpoint(ul/min) 5"() -> (w84:dbl)
        n930 = local read "Pump setpoint(ul/min) 6"() -> (w83:dbl)
        n931 = Build Array(w91, w87, w86, w85, w84, w83) -> (w92:dbl[])
        n932 = Array To Cluster(array=w92) -> (cluster=→"Pump Setpoints Chart":T3)
        n933 = Wait (ms)(milliseconds to wait=u32 5000) -> ()  [unwired: 1 out]
        n934 = local read "Stop"() -> (w88:bool)
      }
      n935 = while {
        stop <- w70 stop-if-true
        n936 = local read "System Error"() -> (w69:bool)
        n937 = Wait (ms)(milliseconds to wait=u32 300) -> ()  [unwired: 1 out]
        n938 = case shown="True" w69 {
          tunnel: [w74 w75] -> w67
          frame False {
            w71 = u16 2 items=["System  Error", "System Running", "System Standby"] ("System Status")
            w72 = u16 1 items=["System  Error", "System Running", "System Standby"] ("System Status")
            n939 = local read "running?"() -> (w73:bool)
            n940 = Select(t=w72, s=w73, f=w71) -> (s? t:f=w74:u16)
          }
          frame True {
            w75 = u16 0 items=["System  Error", "System Running", "System Standby"] ("System Status")
          }
        }
        n941 = local read "Stop"() -> (w70:bool)
        n942 = local write "System Status"(w67) -> ()
      }
      n943 = while {
        tunnel: w61 -> [w76]
        stop <- w82 stop-if-true
        n944 = call-poly <vilib>:"Analog Read.vi"("Analog Channel"=u8 0, "LINX Resource"=w76) -> ("Voltage"=w77:dbl)  [unwired: 6 in, 3 out]
        "Phase_Sensor_voltage" <- w77
        n945 = Wait (ms)(milliseconds to wait=u32 300) -> ()  [unwired: 1 out]
        n946 = Build Array(w77) -> (w79:dbl[])
        n947 = Array To Cluster(array=w79) -> (cluster=→"Phase Sensor Chart":T3)
        n948 = local read "Stop"() -> (w82:bool)
      }
      n949 = while {
        tunnel: w61 -> [w95]
        stop <- w120 stop-if-true
        w102 = 270
        w96 = 600
        w97 = 600
        # "Read Pressure and Flowrate"
        n950 = local read "Stop"() -> (w120:bool)
        n951 = call-poly <vilib>:"Analog Read.vi"("AI Channel(s)"=i32[] [14, 15, 14, 15], "LINX Resource"=w95) -> ("Voltages"=w93:dbl[])  [unwired: 6 in, 3 out]
        n952 = Index Array(array=w93, index=1) -> (element=w116:dbl)
        n953 = Index Array(array=w93, index=0) -> (element=w117:dbl)
        n954 = call-poly <vilib>:"PID Control Input Filter.vi"("input"=w116) -> ("output"=w109:dbl)  [unwired: 4 in]
        n955 = call-poly <vilib>:"PID Control Input Filter.vi"("input"=w117) -> ("output"=w108:dbl)  [unwired: 4 in]
        n956 = Multiply(x=104.96 ("y"), y=w109) -> (x*y=w110:dbl)
        n957 = Multiply(x=104.96 ("y"), y=w108) -> (x*y=w113:dbl)
        n958 = Subtract(x=w110, y=24.077) -> (x-y=w100:dbl)
        n959 = Subtract(x=w113, y=24.077) -> (x-y=w101:dbl)
        n960 = Build Array(w97, w96) -> (w105:i32[])
        n961 = Array To Cluster(array=w105) -> (cluster=→"Flowrate Chart":T4)
        n962 = Build Array(w101, w100) -> (w106:dbl[])
        n963 = local write "Flowrate Sensor 1"(w97) -> ()
        n964 = local write "Flowrate Sensor 2"(w96) -> ()
        n965 = local write "Pressure 1"(w101) -> ()
        n966 = local write "Pressure 2"(w100) -> ()
        n967 = Array To Cluster(array=w106) -> (cluster=→"Pressure Chart":T3)
        n968 = Wait (ms)(milliseconds to wait=u32 500) -> ()  [unwired: 1 out]
        n969 = script code="MATLAB script"("F1"=w97, "F2"=w96, "Pres1"=w101, "Pres2"=w100) -> ()  [unwired: 1 in, 1 out]
        n970 = Greater?(x=w100, y=w102) -> (0:w98:bool)
        n971 = Greater?(x=w101, y=w102) -> (0:w99:bool)
        n972 = case shown="False" w99 {
          frame False {
          }
          frame True {
            w124 = TRUE ("Stop")
            n973 = local write "System Error"(w124) -> ()
            n974 = local write "Stop"(w124) -> ()
            n975 = local write "Error Message"("Pressure Sensor 1 readings above 250psi") -> ()
            n976 = script code="system_error = 1;"() -> ()  [unwired: 1 in, 1 out]
          }
        }
        n977 = case shown="True" w98 {
          frame False {
          }
          frame True {
            w122 = TRUE ("Stop")
            n978 = local write "System Error"(w122) -> ()
            n979 = local write "Error Message"("Pressure Sensor 2 readings above 250psi") -> ()
            n980 = local write "Stop"(w122) -> ()
            n981 = script code="system_error = 1;"() -> ()  [unwired: 1 in, 1 out]
          }
        }
      }
    }
    frame #3 {
      # "Save and close xml and excel file"
      n982 = script code="if exist('xl_file','var') & exist('xlApp','var')\n  xlWorkbook.SaveAs(xl_file);\n  xlWorkbook.Close;\n  xlApp.Quit;\n  xlApp.delete;\nend"() -> ()  [unwired: 1 in, 1 out]
    }
    frame #4 {
      w1319 = string[] ["e", "f", "g", "h", "i", "j"]
      # "End communication to hardware"
      n983 = local read "Syringe_pump?"() -> (w1317:bool)
      n984 = local read "COMM Port:: Harvard Syringe Pump"() -> (w1318:refnum<visa-resource-name>)
      n985 = local read "IR Sensor Device"() -> (w1316:T6)
      n986 = local read "COMM Port :: Milligat Pumps"() -> (w1321:refnum<visa-resource-name>)
      n987 = call <vilib>:"Close.vi"("LINX Resource"=w1315) -> ()  [unwired: 10 in, 1 out]
      n988 = Array Size(array=w1319) -> (size(s)=w1320:i32)
      n989 = case shown="True" w1317 {
        tunnel: w1318 -> [_ w1322]
        frame False {
        }
        frame True {
          n990 = call <instrlib>:"Stop Pump.vi"("VISA resource name"=w1322) -> ()  [unwired: 9 in, 2 out]
        }
      }
      n991 = for {
        N: w1320 -> [_]
        tunnel: w1319 -> [w1323] mode=indexing
        tunnel: w1321 -> [w1324]
        n992 = call "PumpStop.vi"("Pump Address"=w1323, "Pump COMM Port"=w1324) -> ()  [unwired: 9 in, 1 out]
        n993 = Wait (ms)(milliseconds to wait=u32 300) -> ()  [unwired: 1 out]
      }
      n994 = call-poly <vilib>:"NI-845x Close Reference.vi"("device reference"=w1316) -> ()  [unwired: 10 in, 1 out]
    }
    frame #5 {
      # "Display Error Messages if necessary"
      n995 = local read "Error Message"() -> (w1326:string)
      n996 = One Button Dialog(message=w1326) -> ()  [unwired: 1 in, 1 out]
    }
  }
